vi "Multi U-Link DAQ Single value.vi"() -> ()   [LabVIEW 2017]
uses:
  Type Def/Data.ctl
  <vilib>/Analysis/NI_AALBase.lvlib
panel:
  out "Energie IR mean":dbl caption="moyenne" format="%g"
  out "Energie IR variance":dbl caption="variance" format="%g"
  out "Energie IR max":dbl caption="max" format="%#_5g"
  out "Energie IR min":dbl caption="min"
  out "Puissance depolar mean":dbl caption="moyenne" format="%g"
  out "Puissance depolar variance":dbl caption="variance" format="%g"
  out "Puissance depolar max":dbl caption="max" format="%#_5g"
  out "Puissance depolar min":dbl caption="min" format="%#_5g"
  out "Energie UV mean":dbl caption="moyenne" format="%g"
  out "Energie UV variance":dbl caption="variance" format="%g"
  out "Energie UV max":dbl caption="max" format="%#_5g"
  out "Energie UV min":dbl caption="min" format="%#_5g"
  out "Energie UV rapport":dbl caption="rapport" format="%#_5g"
  out "Puissance depolar rapport":dbl caption="rapport" format="%#_5g"
  out "Energie IR rapport":dbl caption="rapport" format="%#_5g"
  out "Chaîne":string="Energie UV"
  out "Chaîne 2":string="Puissance depolar"
  out "Chaîne 3":string="Energie IR"
  out "sortie d'erreur":errorcluster caption="Sortie d'erreur"
  in  "stop":bool
  out "Energie IR value":dbl format="%#_4f"
  out "Energie IR graph":dbl(graph)
  out "Puissance depolar value":dbl format="%#_4f"
  out "Puissance depolar graph":dbl(graph)
  out "Energie IR table":dbl[](array[numeric])
  out "Energie IR table (1sec)":dbl[](array[numeric])
  out "Puissance depolar table":dbl[](array[numeric])
  out "Energie UV value":dbl format="%#_4f"
  out "Energie UV graph":dbl(graph)
  out "Energie UV table":dbl[](array[numeric])
  out "Energie UV table(1sec)":dbl[](array[numeric])
  out "Taux depolar value":dbl format="%#_4f"
  out "taux depolar graph":dbl(graph)
  out "Puissance depolar table (stats)":dbl[][](array[numeric])
  out "Energie IR table (stats)":dbl[][](array[numeric])
  out "Taux depolar indicator":u32(colorbox)=16777222
  out "Puissance depolar table (1sec)":dbl[](array[numeric])
  out "Energie UV table (stats)":dbl[][](array[numeric])
  out "timer 1sec":bool
  out "timer 12sec":bool
  in  "1sec":bool
  in  "12sec":bool
  out "index 1sec":i32
  out "index 12sec":i32
  out "Chaîne 4":string="Energie UV (mJ)"
  out "Chaîne 5":string="Energie IR (mJ)"
  out "Chaîne 6":string="Puissance depolar (W)"
  out "Chaîne 7":string="Taux depolar"
  out "Update":string="Initialization : matching U-Link ports, creating data file"
  in  "Start acquisition":bool
  in  "Commande onglets":T1(tab)
  out "Ressource VISA (Energie UV)":refnum<visa-resource-name>
  in  "Wavelength (nm) (Energie UV)":u32=355
  in  "Offset (Energie UV)":sgl
  in  "Multiplier (Energie UV)":sgl=1.0
  in  "Trigger Level (% of Scale) (Energie UV)":dbl=2.0 min=0.1 max=99.9 step=0.1 format="%_3f"
  in  "Auto Scale (Energie UV)":bool=TRUE
  out "File name (Energie UV)":string="data.csv"
  in  "Scale (Watt or Joule) (Energie UV)":i32(ring) items=["1 pico", "3 pico", "10 pico", "30 pico", "100 pico", "300 pico", "1 nano", "3 nano", "10 nano", "30 nano", "100 nano", "300 nano", "1 micro", "3 micro", "10 micro", "30 micro", "100 micro", "300 micro", "1 milli", "3 milli", "10 milli", "30 milli", "100 milli", "300 milli", "1", "3", "10", "30", "100", "300", "1 kilo", "3 kilo", "10 kilo", "30 kilo", "100 kilo", "300 kilo", "1 mega", "3 mega", "10 mega", "30 mega", "100 mega", "300 mega"]
  out "Ressource VISA (Puissance depolar)":refnum<visa-resource-name>
  in  "Offset (Puissance depolar)":sgl
  in  "Wavelength (nm) (Puissance depolar)":u32=1064
  in  "Multiplier (Puissance depolar)":sgl=1.0
  in  "Trigger Level (% of Scale) (Puissance depolar)":dbl=2.0 min=0.1 max=99.9 step=0.1 format="%_3f"
  in  "Auto Scale (Puissance depolar)":bool=TRUE
  out "File name (Puissance depolar)":string="data.csv"
  in  "Scale (Watt or Joule) (Puissance depolar)":u16(ring) items=["1 pico", "3 pico", "10 pico", "30 pico", "100 pico", "300 pico", "1 nano", "3 nano", "10 nano", "30 nano", "100 nano", "300 nano", "1 micro", "3 micro", "10 micro", "30 micro", "100 micro", "300 micro", "1 milli", "3 milli", "10 milli", "30 milli", "100 milli", "300 milli", "1", "3", "10", "30", "100", "300", "1 kilo", "3 kilo", "10 kilo", "30 kilo", "100 kilo", "300 kilo", "1 mega", "3 mega", "10 mega", "30 mega", "100 mega", "300 mega"]
  out "Ressource VISA (Energie IR)":refnum<visa-resource-name>
  in  "Wavelength (nm) (Energie IR)":u32=1064
  in  "Offset (Energie IR)":sgl
  in  "Multiplier (Energie IR)":sgl=1.0
  in  "Trigger Level (% of Scale) (Energie IR)":dbl=2.0 min=0.1 max=99.9 step=0.1 format="%_3f"
  out "File name (Energie IR)":string="data.csv"
  in  "Scale (Watt or Joule) (Energie IR)":u16(ring) items=["1 pico", "3 pico", "10 pico", "30 pico", "100 pico", "300 pico", "1 nano", "3 nano", "10 nano", "30 nano", "100 nano", "300 nano", "1 micro", "3 micro", "10 micro", "30 micro", "100 micro", "300 micro", "1 milli", "3 milli", "10 milli", "30 milli", "100 milli", "300 milli", "1", "3", "10", "30", "100", "300", "1 kilo", "3 kilo", "10 kilo", "30 kilo", "100 kilo", "300 kilo", "1 mega", "3 mega", "10 mega", "30 mega", "100 mega", "300 mega"]
  in  "Auto Scale (Energie IR)":bool
  out "error IO":errorcluster
  out "COM Port table":refnum<visa-resource-name>[](array[refnum])
  out "COM Port (Energie IR)":i64
  out "COM Port (Puissance depolar)":i64
  out "COM port (Energie UV)":i64
  out "User file contents Energie UV":dbl[](array[numeric])
  out "User file contents Energie IR":dbl[](array[numeric])
  out "User file contents Puissance depolar":dbl[](array[numeric])
  out "error?":bool caption="erreur ?"
  out "file path":path
  out "sortie d'erreur 3":errorcluster caption="sortie d'erreur"
  out "sortie d'erreur 2":errorcluster caption="sortie d'erreur"
  out "Energie UV file (1sec)":refnum<file>
  out "Energie UV file (stats)":refnum<file>
  out "Puissance depolar file (1sec)":refnum<file>
  out "Puissance depolar file (stats)":refnum<file>
  out "Energie IR file (1sec)":refnum<file>
  out "Energie IR file (stats)":refnum<file>
  in  "Bouton Accueil":bool
  out "chaîne de date/heure":string
  out "valeur de l'horloge en ms":u32
  out "Time":string
  out "stop?":bool=TRUE
  out "Tableau Puissance depolar":dbl[](array[numeric])
  out "Tableau UV":dbl[](array[numeric])
  out "Tableau IR":dbl[](array[numeric])
  out "taille UV":dbl format="%.2f"
  out "taille Pd":dbl format="%.2f"
  out "taille IR":dbl format="%.2f"
  out "12sec UV":bool
  out "12sec Pd":bool
  out "12sec IR":bool
  out "stop UV":bool
  out "stop Pd":bool
  out "stop IR":bool
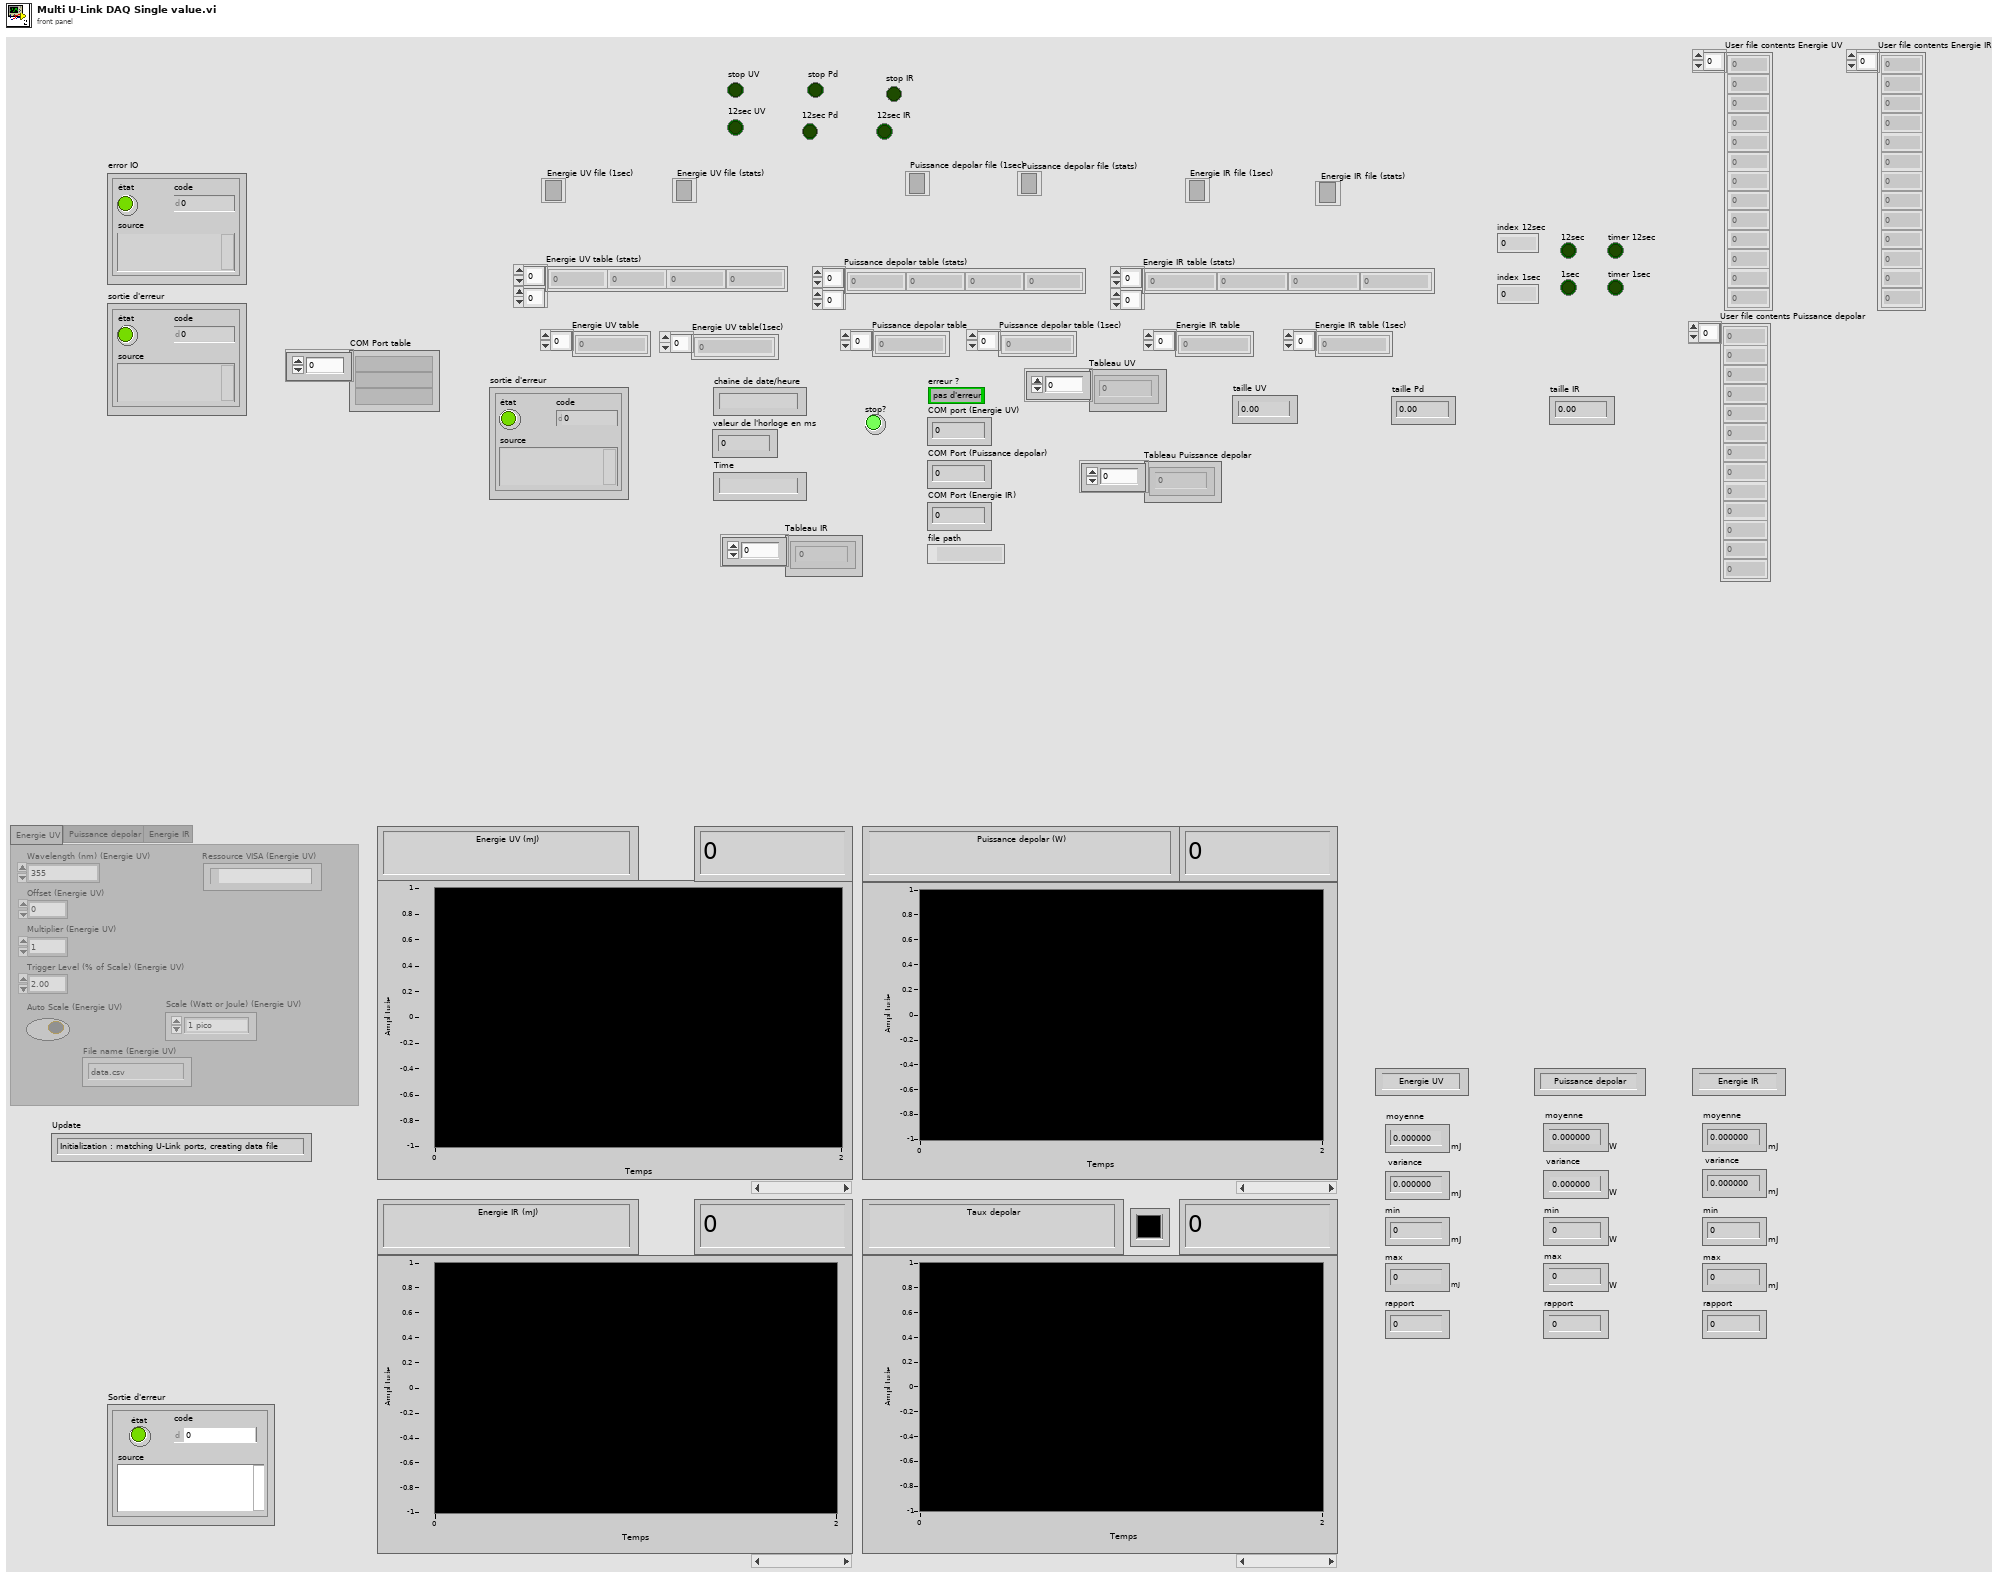
[diagram p1: front panel]
types:
  T1 = enum32{"Energie UV", "Puissance depolar", "Energie IR"}
  T2 = enum8{"Enabled", "Disabled", "Disabled and Grayed Out"}
  T3 = typedef "Data.ctl" = cluster{enum16{"Init", "Read", "Stop", "12sec"}, "Data":dbl}
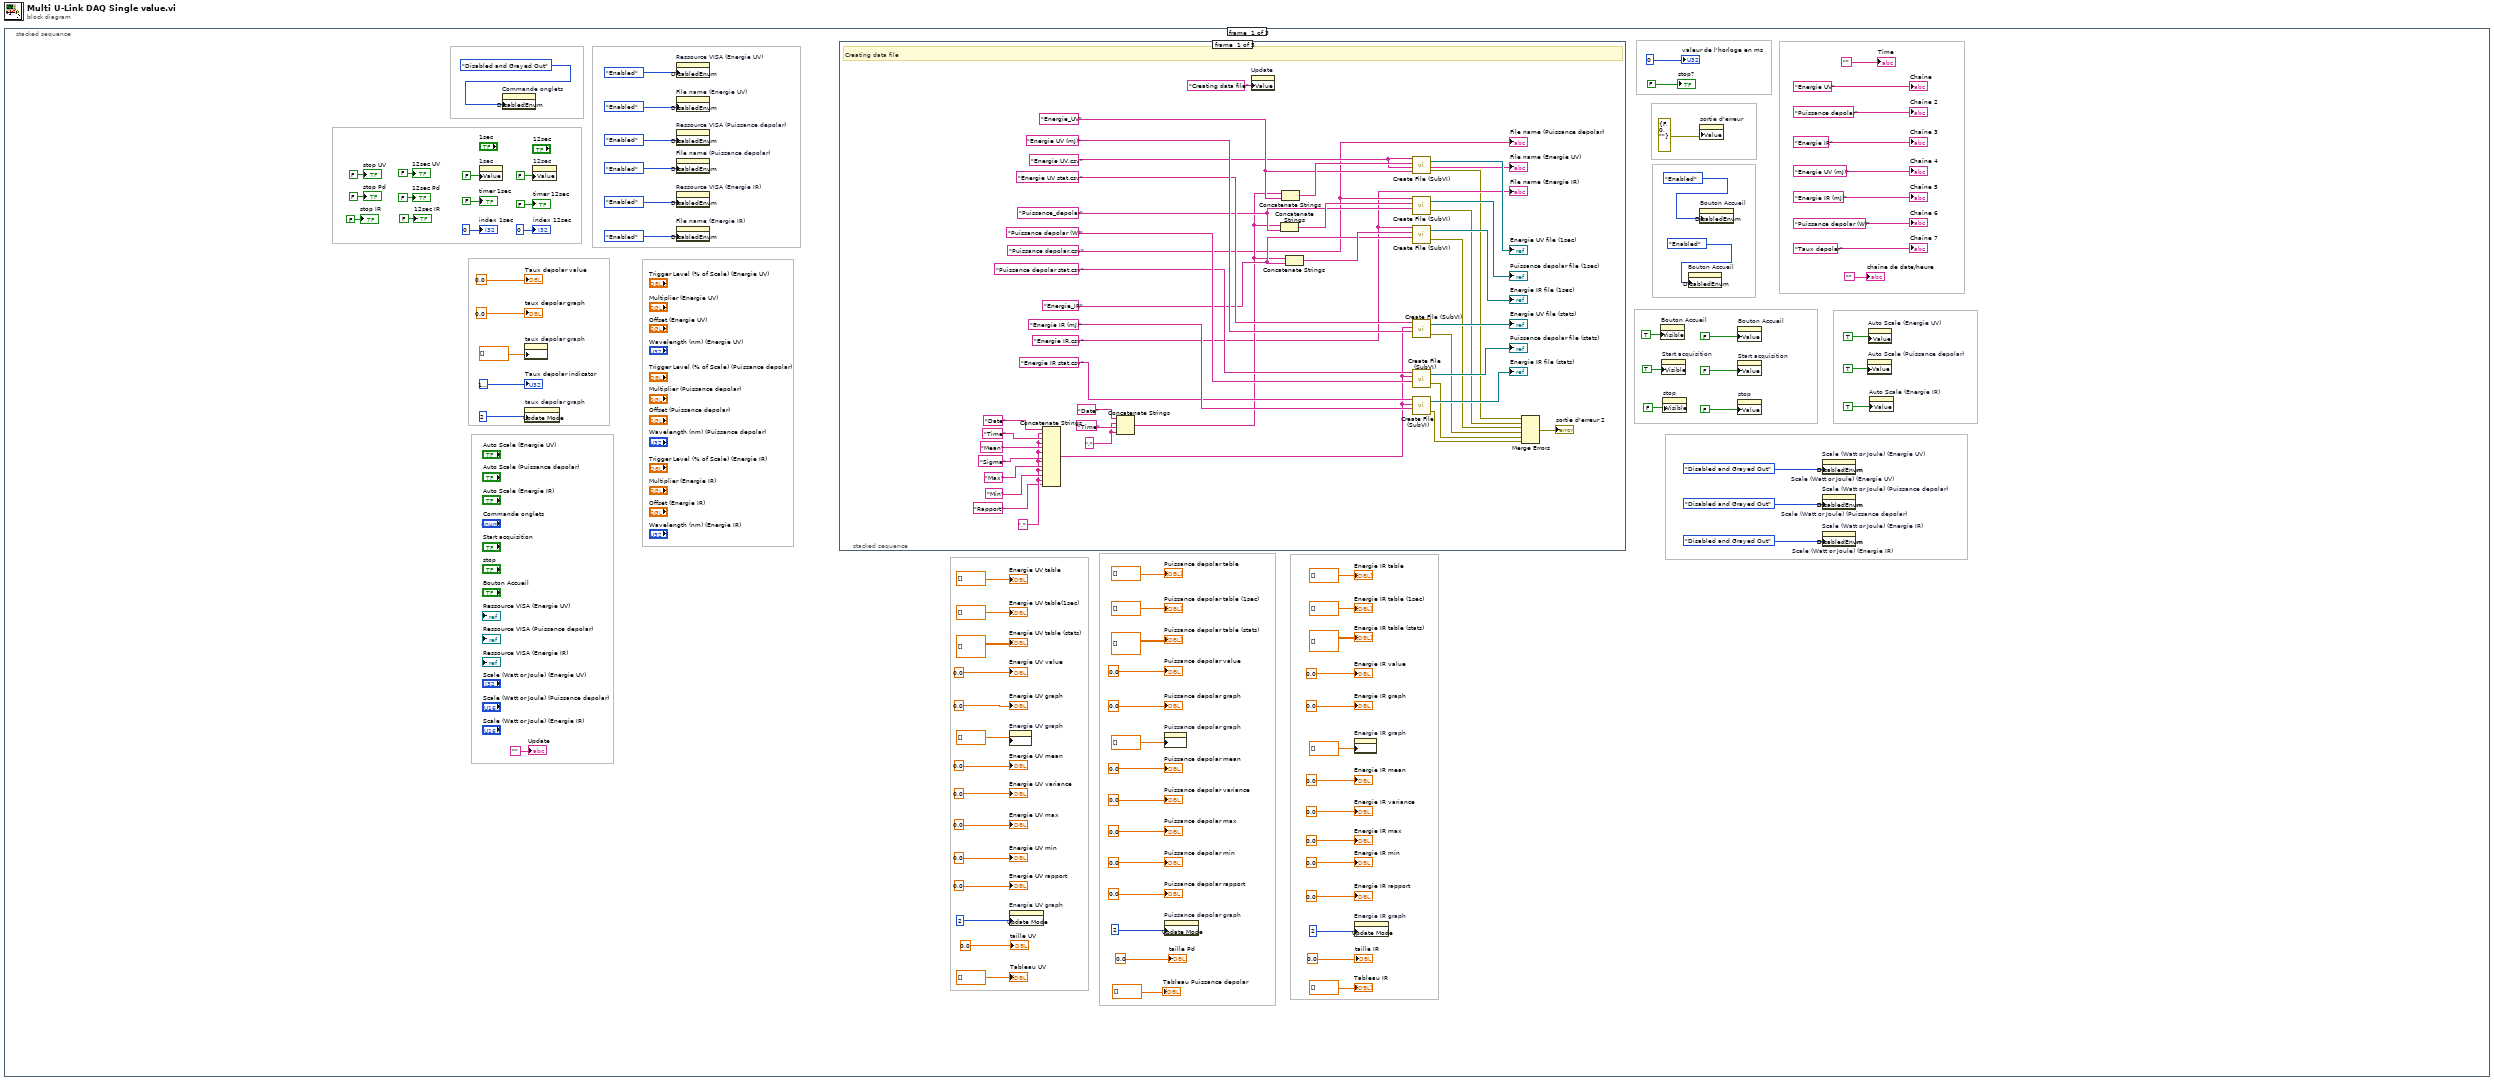
[diagram p0: block diagram]
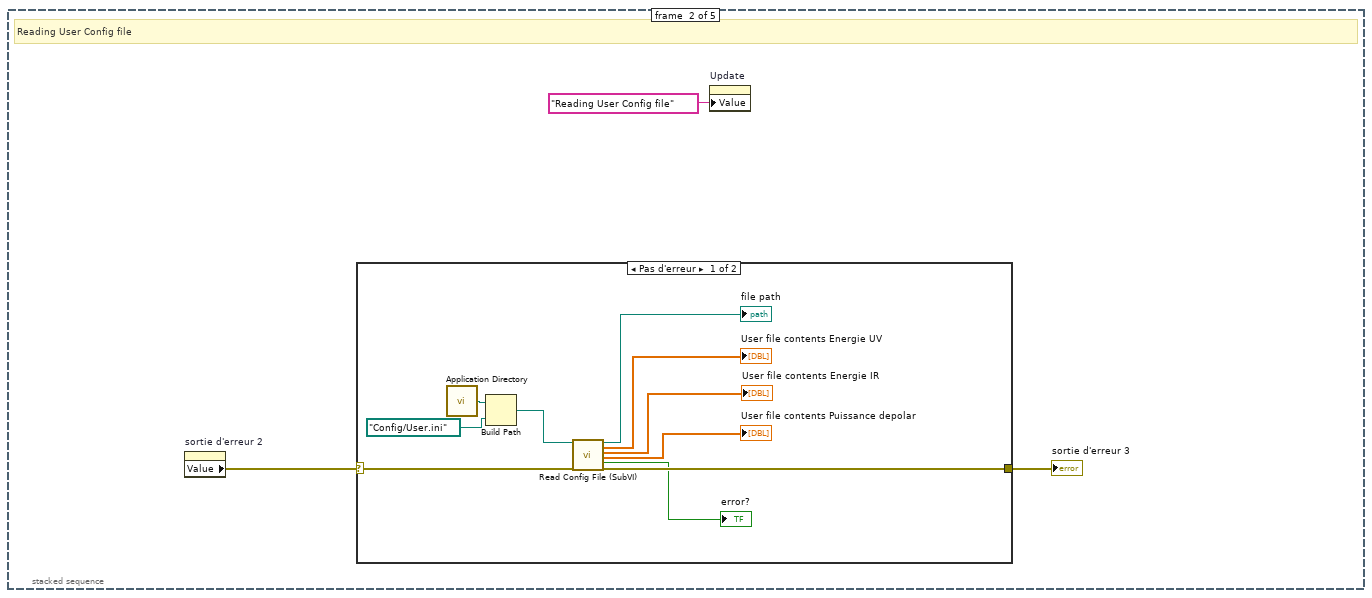
[diagram p2: hidden frame]
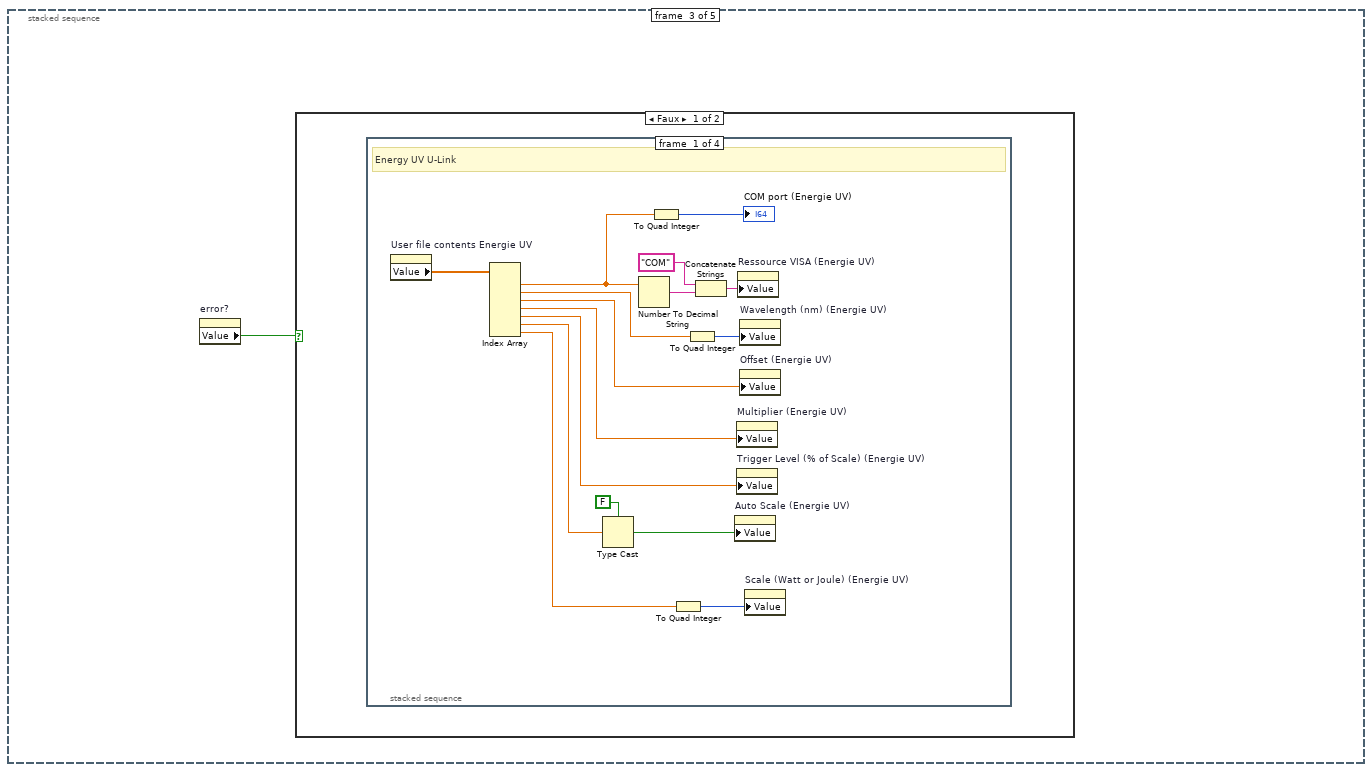
[diagram p4: hidden frame]
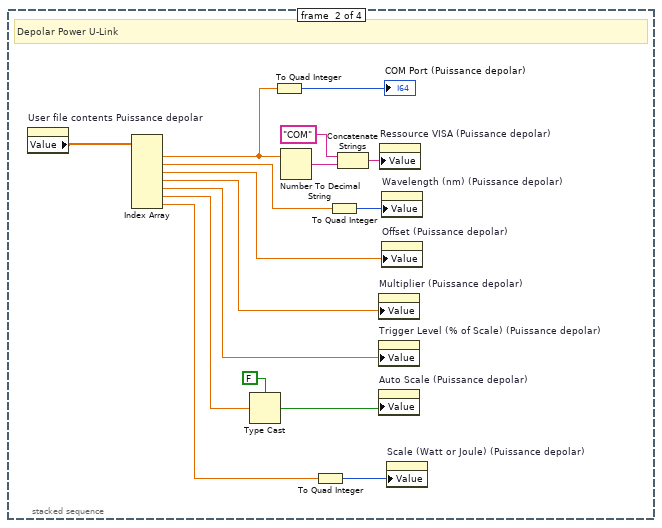
[diagram p5: hidden frame]
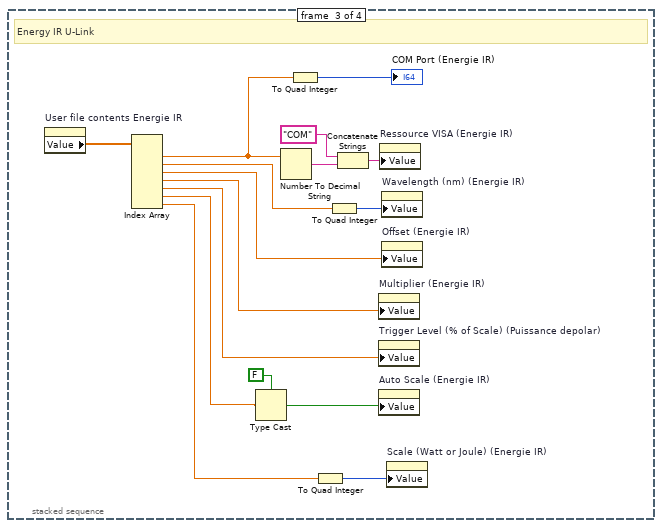
[diagram p6: hidden frame]
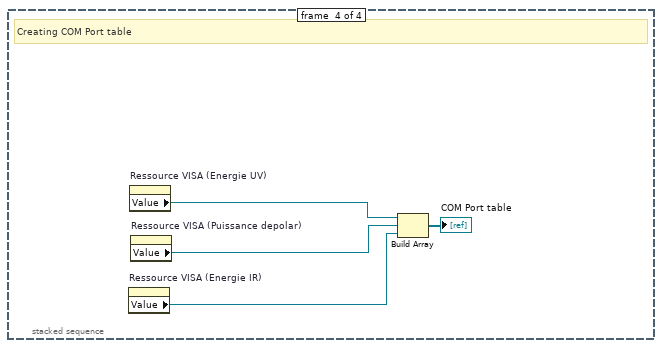
[diagram p7: hidden frame]
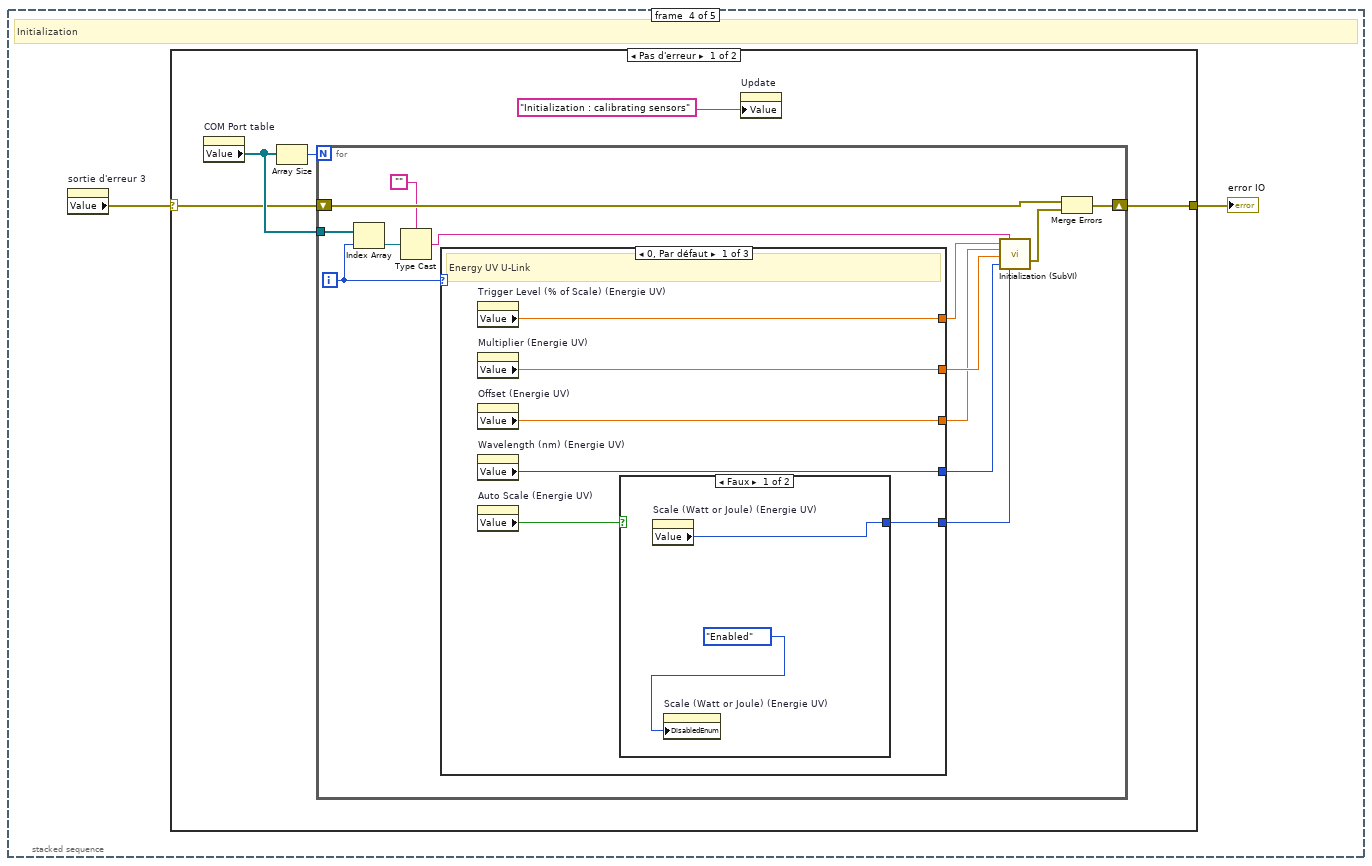
[diagram p9: hidden frame]
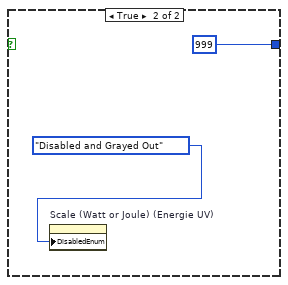
[diagram p10: hidden frame]
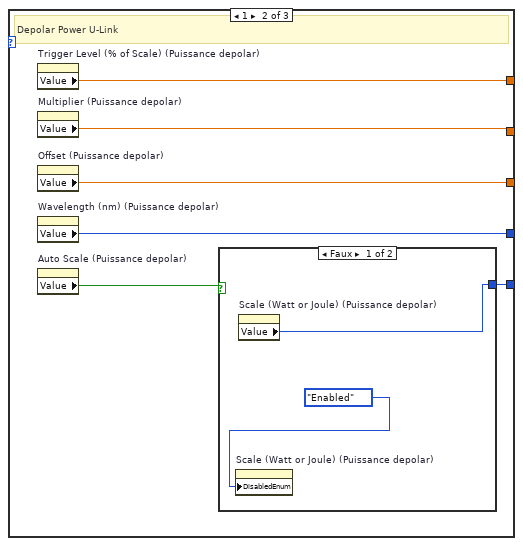
[diagram p11: hidden frame]
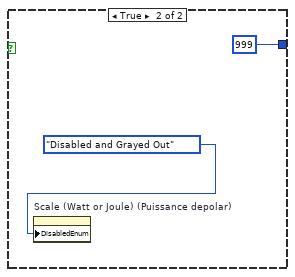
[diagram p12: hidden frame]
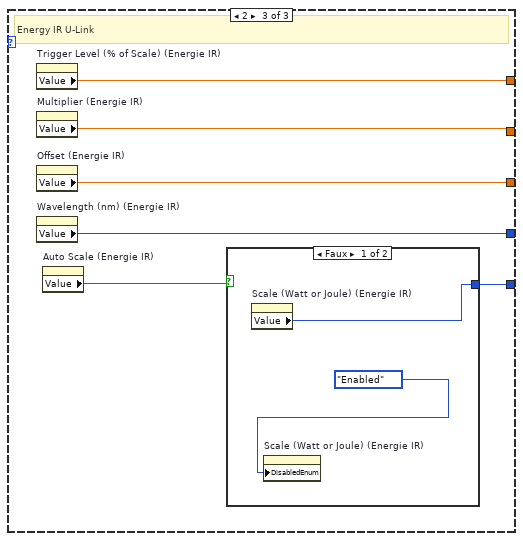
[diagram p13: hidden frame]
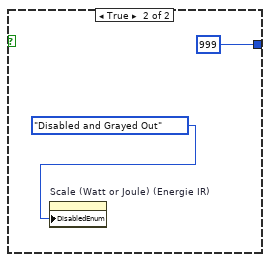
[diagram p14: hidden frame]
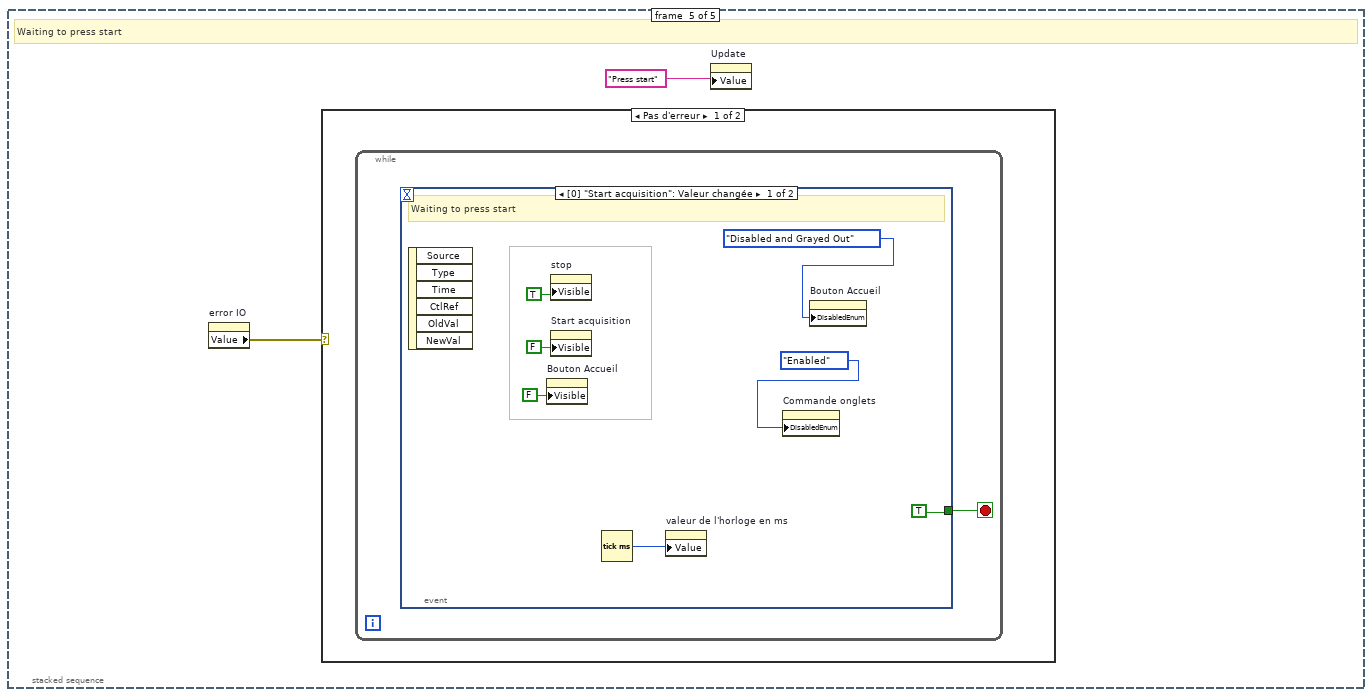
[diagram p16: hidden frame]
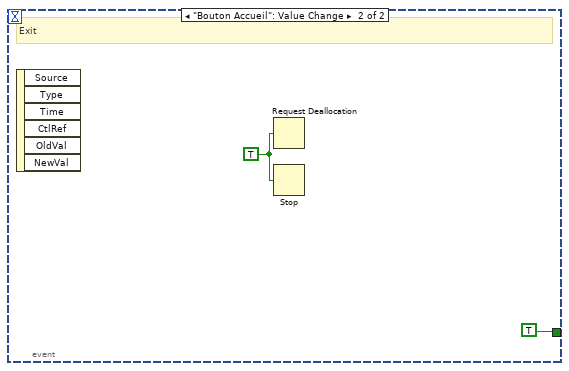
[diagram p17: hidden frame]
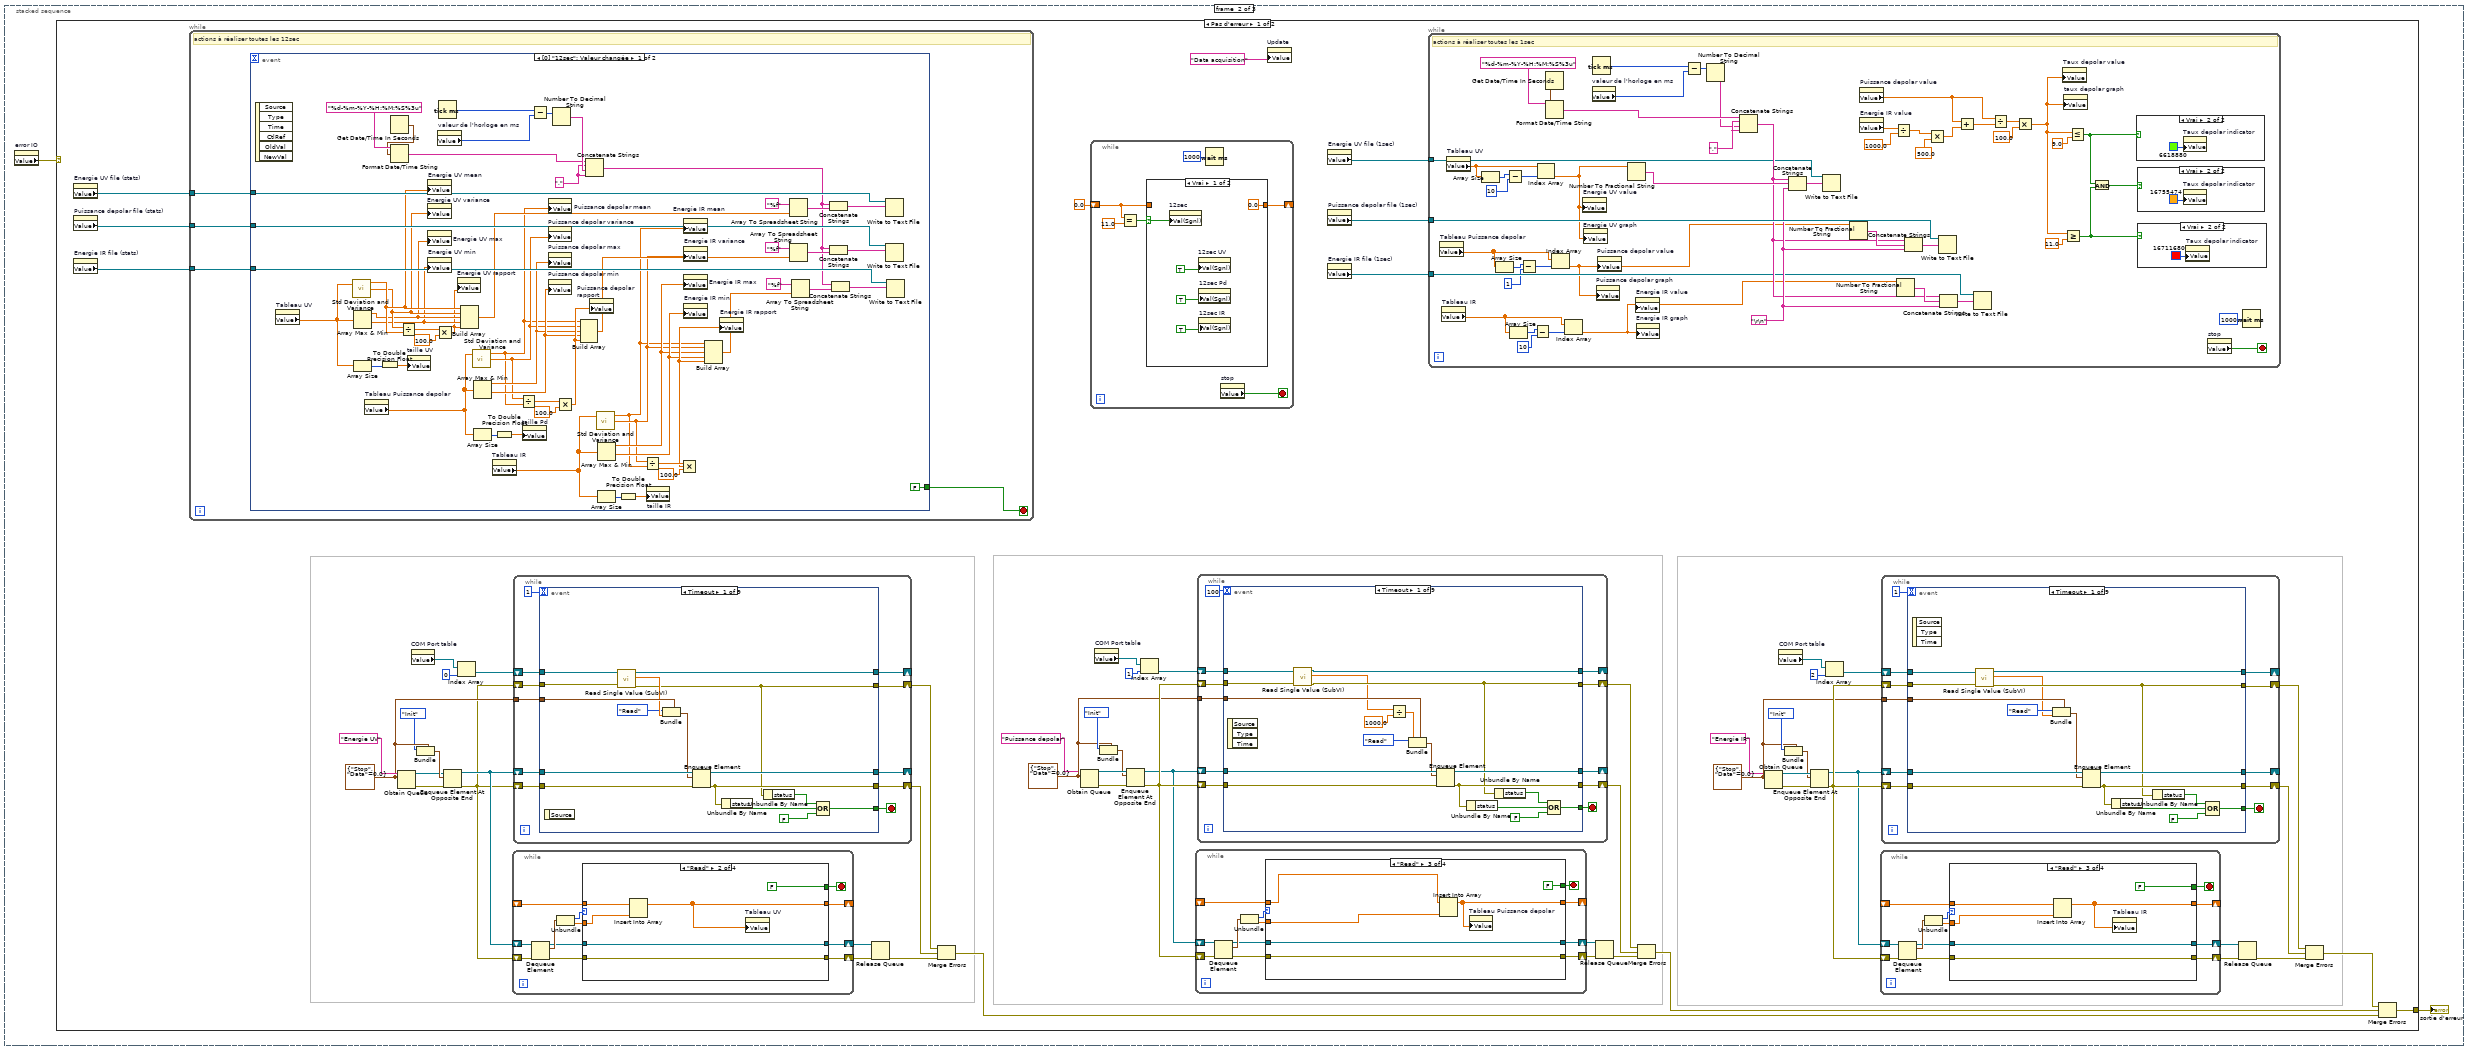
[diagram p19: hidden frame]
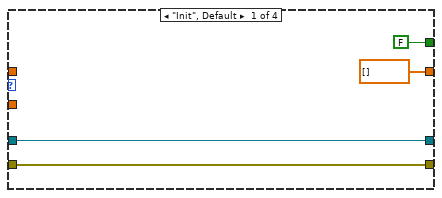
[diagram p20: hidden frame]
diagram:
  n1 = stacked-sequence {
    frame #0 {
      n2 = property on="1sec" class="Bool (strict)"("Value"=FALSE ("1sec")) -> ()  [unwired: 2 in, 2 out]
      n3 = property on="Commande onglets" class="Onglet (strict)"("DisabledEnum"=T2."Disabled and Grayed Out" ("Désactivé")) -> ()  [unwired: 2 in, 2 out]
      n4 = property on="taux depolar graph" class="GraphDér (strict)"("History Data"=dbl[] [] ("Données d'historique")) -> ()  [unwired: 2 in, 2 out]
      n5 = property on="taux depolar graph" class="GraphDér (strict)"("Update Mode"=u8 2 ("Mode de rafraîchissement")) -> ()  [unwired: 2 in, 2 out]
      n6 = property on="12sec" class="Bool (strict)"("Value"=FALSE ("12sec")) -> ()  [unwired: 2 in, 2 out]
      n7 = property on="Ressource VISA (Energie UV)" class="NomVISA"("DisabledEnum"=T2."Enabled" ("Désactivé")) -> ()  [unwired: 2 in, 2 out]
      n8 = property on="File name (Energie UV)" class="Ch"("DisabledEnum"=T2."Enabled" ("Désactivé")) -> ()  [unwired: 2 in, 2 out]
      n9 = property on="Ressource VISA (Puissance depolar)" class="NomVISA"("DisabledEnum"=T2."Enabled" ("Désactivé")) -> ()  [unwired: 2 in, 2 out]
      n10 = property on="File name (Puissance depolar)" class="Ch"("DisabledEnum"=T2."Enabled" ("Désactivé")) -> ()  [unwired: 2 in, 2 out]
      n11 = property on="Ressource VISA (Energie IR)" class="NomVISA"("DisabledEnum"=T2."Enabled" ("Désactivé")) -> ()  [unwired: 2 in, 2 out]
      n12 = property on="File name (Energie IR)" class="Ch"("DisabledEnum"=T2."Enabled" ("Désactivé")) -> ()  [unwired: 2 in, 2 out]
      n13 = stacked-sequence {
        frame #0 {
          w114 = ","
          w104 = ","
          w105 = "Energie IR.csv" ("file name 2")
          w109 = "Energie_IR" ("data name")
          w106 = "Puissance depolar.csv" ("file name 2")
          w111 = "Puissance_depolar" ("data name")
          w107 = "Energie UV.csv" ("file name")
          w116 = "Energie_UV" ("data name")
          # "Creating data file"
          n14 = Concatenate Strings("Date", w104, "Time", w104, "Mean", w104, "Sigma", w104, "Max", w104, "Min", w104, "Rapport" ("chaîne")) -> (w120:string)
          n15 = Concatenate Strings("Date", w114, "Time", w114) -> (w108:string)
          n16 = property on="Update" class="Ch"("Value"="Creating data file" ("Étiquette.Texte")) -> ()  [unwired: 2 in, 2 out]
          n17 = Concatenate Strings(w108, w111) -> (w112:string)
          n18 = Concatenate Strings(w108, w116) -> (w117:string)
          n19 = Concatenate Strings(w108, w109) -> (w110:string)
          n20 = call "Create File (SubVI).vi"("headers"=w116, "data name"=w117, "file name"=w107) -> ("error out"=w97:errorcluster, "Byte Stream File out"=→"Energie UV file (1sec)":refnum<file>)  [unwired: 1 in]
          n21 = call "Create File (SubVI).vi"("headers"=w111, "data name"=w112, "file name"=w106) -> ("error out"=w98:errorcluster, "Byte Stream File out"=→"Puissance depolar file (1sec)":refnum<file>)  [unwired: 1 in]
          n22 = call "Create File (SubVI).vi"("headers"=w109, "data name"=w110, "file name"=w105) -> ("error out"=w99:errorcluster, "Byte Stream File out"=→"Energie IR file (1sec)":refnum<file>)  [unwired: 1 in]
          n23 = call "Create File (SubVI).vi"("headers"="Energie UV (mJ)" ("data name"), "data name"=w120, "file name"="Energie UV stat.csv") -> ("error out"=w100:errorcluster, "Byte Stream File out"=→"Energie UV file (stats)":refnum<file>)  [unwired: 1 in]
          n24 = call "Create File (SubVI).vi"("headers"="Puissance depolar (W)" ("data name"), "data name"=w120, "file name"="Puissance depolar stat.csv" ("file name 2")) -> ("error out"=w101:errorcluster, "Byte Stream File out"=→"Puissance depolar file (stats)":refnum<file>)  [unwired: 1 in]
          n25 = call "Create File (SubVI).vi"("headers"="Energie IR (mJ)" ("data name"), "data name"=w120, "file name"="Energie IR stat.csv" ("file name 2")) -> ("error out"=w102:errorcluster, "Byte Stream File out"=→"Energie IR file (stats)":refnum<file>)  [unwired: 1 in]
          n26 = Merge Errors(w97, w98, w99, w100, w101, w102) -> (→"sortie d'erreur 2":errorcluster)
          "File name (Energie UV)" <- w107
          "File name (Puissance depolar)" <- w106
          "File name (Energie IR)" <- w105
        }
        frame #1 {
          # "Reading User Config file"
          n27 = property on="sortie d'erreur 2" class="Clust (strict)"() -> ("Value"=w141:errorcluster)  [unwired: 2 in, 2 out]
          n28 = case shown="Pas d'erreur" w141 {
            selector: w141 -> [w150 w152]
            tunnel: [w151 w152] -> w140
            frame No Error {
              n29 = call <vilib>:"Application Directory.vi"() -> ("Application Directory"=w146:path)
              n30 = Build Path(base path=w146, name or relative path=path "Config/User.ini") -> (appended path=w144:path)
              n31 = call "Read Config File (SubVI).vi"("configuration file path"=w144, "entrée d'erreur (pas d'erreur)"=w150) -> ("file path"=→"file path":path, "User file contents Energie UV"=→"User file contents Energie UV":dbl[], "User file contents Energie IR"=→"User file contents Energie IR":dbl[], "User file contents Puissance depolar"=→"User file contents Puissance depolar":dbl[], "error?"=→"error?":bool, "sortie d'erreur"=w151:errorcluster)  [unwired: 12 in]
            }
            frame Error {
            }
          }
          "sortie d'erreur 3" <- w140
          n32 = property on="Update" class="Ch"("Value"="Reading User Config file" ("Étiquette.Texte")) -> ()  [unwired: 2 in, 2 out]
        }
        frame #2 {
          n33 = property on="error?" class="Bool (strict)"() -> ("Value"=w153:bool)  [unwired: 2 in, 2 out]
          n34 = case shown="Faux" w153 {
            frame False {
              n35 = stacked-sequence {
                frame #0 {
                  # "Energy UV U-Link"
                  n36 = property on="User file contents Energie UV" class="Tabl (strict)"() -> ("Value"=w154:dbl[])  [unwired: 2 in, 2 out]
                  n37 = Index Array(array=w154) -> (element #1=w166:dbl, element #2=w165:dbl, element #3=w163:dbl, element #4=w162:dbl, element #5=w157:dbl, element #6=w156:dbl, element #7=w155:dbl)  [unwired: 7 in]
                  n38 = Type Cast(type=FALSE, x=w156) -> (*(type *) &x=w159:bool)
                  n39 = Number To Decimal String(number=w166) -> (decimal integer string=w168:string)  [unwired: 1 in]
                  n40 = To Quad Integer(1:w166) -> (0:→"COM port (Energie UV)":i64)
                  n41 = To Quad Integer(1:w155) -> (0:w161:i64)
                  n42 = To Quad Integer(1:w165) -> (0:w164:i64)
                  n43 = Concatenate Strings("COM" ("string"), w168) -> (w167:string)
                  n44 = property on="Auto Scale (Energie UV)" class="Bool (strict)"("Value"=w159) -> ()  [unwired: 2 in, 2 out]
                  n45 = property on="Multiplier (Energie UV)" class="NumNb (strict)"("Value"=w162) -> ()  [unwired: 2 in, 2 out]
                  n46 = property on="Trigger Level (% of Scale) (Energie UV)" class="NumNb (strict)"("Value"=w157) -> ()  [unwired: 2 in, 2 out]
                  n47 = property on="Ressource VISA (Energie UV)" class="NomVISA"("Value"=w167) -> ()  [unwired: 2 in, 2 out]
                  n48 = property on="Wavelength (nm) (Energie UV)" class="NumNb (strict)"("Value"=w164) -> ()  [unwired: 2 in, 2 out]
                  n49 = property on="Offset (Energie UV)" class="NumNb (strict)"("Value"=w163) -> ()  [unwired: 2 in, 2 out]
                  n50 = property on="Scale (Watt or Joule) (Energie UV)" class="MDér (strict)"("Value"=w161) -> ()  [unwired: 2 in, 2 out]
                }
                frame #1 {
                  # "Depolar Power U-Link"
                  n51 = property on="User file contents Puissance depolar" class="Tabl (strict)"() -> ("Value"=w176:dbl[])  [unwired: 2 in, 2 out]
                  n52 = Index Array(array=w176) -> (element #1=w182:dbl, element #2=w181:dbl, element #3=w179:dbl, element #4=w178:dbl, element #5=w172:dbl, element #6=w171:dbl, element #7=w170:dbl)  [unwired: 7 in]
                  n53 = Type Cast(type=FALSE, x=w171) -> (*(type *) &x=w173:bool)
                  n54 = To Quad Integer(1:w182) -> (0:→"COM Port (Puissance depolar)":i64)
                  n55 = Number To Decimal String(number=w182) -> (decimal integer string=w184:string)  [unwired: 1 in]
                  n56 = To Quad Integer(1:w170) -> (0:w177:i64)
                  n57 = To Quad Integer(1:w181) -> (0:w180:i64)
                  n58 = Concatenate Strings("COM" ("string"), w184) -> (w183:string)
                  n59 = property on="Multiplier (Puissance depolar)" class="NumNb (strict)"("Value"=w178) -> ()  [unwired: 2 in, 2 out]
                  n60 = property on="Trigger Level (% of Scale) (Puissance depolar)" class="NumNb (strict)"("Value"=w172) -> ()  [unwired: 2 in, 2 out]
                  n61 = property on="Auto Scale (Puissance depolar)" class="Bool (strict)"("Value"=w173) -> ()  [unwired: 2 in, 2 out]
                  n62 = property on="Ressource VISA (Puissance depolar)" class="NomVISA"("Value"=w183) -> ()  [unwired: 2 in, 2 out]
                  n63 = property on="Wavelength (nm) (Puissance depolar)" class="NumNb (strict)"("Value"=w180) -> ()  [unwired: 2 in, 2 out]
                  n64 = property on="Offset (Puissance depolar)" class="NumNb (strict)"("Value"=w179) -> ()  [unwired: 2 in, 2 out]
                  n65 = property on="Scale (Watt or Joule) (Puissance depolar)" class="MDér (strict)"("Value"=w177) -> ()  [unwired: 2 in, 2 out]
                }
                frame #2 {
                  # "Energy IR U-Link"
                  n66 = property on="User file contents Energie IR" class="Tabl (strict)"() -> ("Value"=w192:dbl[])  [unwired: 2 in, 2 out]
                  n67 = Index Array(array=w192) -> (element #1=w198:dbl, element #2=w197:dbl, element #3=w195:dbl, element #4=w194:dbl, element #5=w188:dbl, element #6=w187:dbl, element #7=w186:dbl)  [unwired: 7 in]
                  n68 = Type Cast(type=FALSE, x=w187) -> (*(type *) &x=w190:bool)
                  n69 = Number To Decimal String(number=w198) -> (decimal integer string=w200:string)  [unwired: 1 in]
                  n70 = To Quad Integer(1:w198) -> (0:→"COM Port (Energie IR)":i64)
                  n71 = To Quad Integer(1:w186) -> (0:w193:i64)
                  n72 = To Quad Integer(1:w197) -> (0:w196:i64)
                  n73 = Concatenate Strings("COM" ("string"), w200) -> (w199:string)
                  n74 = property on="Multiplier (Energie IR)" class="NumNb (strict)"("Value"=w194) -> ()  [unwired: 2 in, 2 out]
                  n75 = property on="Trigger Level (% of Scale) (Puissance depolar)" class="NumNb (strict)"("Value"=w188) -> ()  [unwired: 2 in, 2 out]
                  n76 = property on="Auto Scale (Energie IR)" class="Bool (strict)"("Value"=w190) -> ()  [unwired: 2 in, 2 out]
                  n77 = property on="Ressource VISA (Energie IR)" class="NomVISA"("Value"=w199) -> ()  [unwired: 2 in, 2 out]
                  n78 = property on="Wavelength (nm) (Energie IR)" class="NumNb (strict)"("Value"=w196) -> ()  [unwired: 2 in, 2 out]
                  n79 = property on="Offset (Energie IR)" class="NumNb (strict)"("Value"=w195) -> ()  [unwired: 2 in, 2 out]
                  n80 = property on="Scale (Watt or Joule) (Energie IR)" class="MDér (strict)"("Value"=w193) -> ()  [unwired: 2 in, 2 out]
                }
                frame #3 {
                  # "Creating COM Port table"
                  n81 = property on="Ressource VISA (Energie IR)" class="NomVISA"() -> ("Value"=w205:refnum<visa-resource-name>)  [unwired: 2 in, 2 out]
                  n82 = property on="Ressource VISA (Energie UV)" class="NomVISA"() -> ("Value"=w203:refnum<visa-resource-name>)  [unwired: 2 in, 2 out]
                  n83 = property on="Ressource VISA (Puissance depolar)" class="NomVISA"() -> ("Value"=w204:refnum<visa-resource-name>)  [unwired: 2 in, 2 out]
                  n84 = Build Array(w203, w204, w205) -> (→"COM Port table":refnum<visa-resource-name>[])
                }
              }
            }
            frame True {
            }
          }
        }
        frame #3 {
          # "Initialization"
          n85 = property on="sortie d'erreur 3" class="Clust (strict)"() -> ("Value"=w206:errorcluster)  [unwired: 2 in, 2 out]
          n86 = case shown="Pas d'erreur" w206 {
            selector: w206 -> [w208 w256]
            tunnel: [w211 w256] -> w207
            frame No Error {
              n87 = property on="COM Port table" class="Tabl (strict)"() -> ("Value"=w209:refnum<visa-resource-name>[])  [unwired: 2 in, 2 out]
              n88 = Array Size(array=w209) -> (size(s)=w210:i32)
              n89 = for {
                N: w210 -> [_]
                shift-right: [w219] -> w211
                shift-left: w208 -> [w218]
                tunnel: w209 -> [w213]
                i -> [w214]
                n90 = Index Array(array=w213, index=w214) -> (element=w216:refnum<visa-resource-name>)
                n91 = Type Cast(type="", x=w216) -> (*(type *) &x=w217:string)
                n92 = case shown="0, Par défaut" w214 {
                  tunnel: [w231 w238 w248] -> w225
                  tunnel: [w228 w239 w249] -> w223
                  tunnel: [w230 w240 w250] -> w224
                  tunnel: [w229 w241 w251] -> w222
                  tunnel: [w227 w237 w247] -> w221
                  frame 0, Default {
                    # "Energy UV U-Link"
                    n93 = property on="Trigger Level (% of Scale) (Energie UV)" class="NumNb (strict)"() -> ("Value"=w229:dbl)  [unwired: 2 in, 2 out]
                    n94 = property on="Multiplier (Energie UV)" class="NumNb (strict)"() -> ("Value"=w230:sgl)  [unwired: 2 in, 2 out]
                    n95 = property on="Offset (Energie UV)" class="NumNb (strict)"() -> ("Value"=w228:sgl)  [unwired: 2 in, 2 out]
                    n96 = property on="Wavelength (nm) (Energie UV)" class="NumNb (strict)"() -> ("Value"=w231:u32)  [unwired: 2 in, 2 out]
                    n97 = property on="Auto Scale (Energie UV)" class="Bool (strict)"() -> ("Value"=w226:bool)  [unwired: 2 in, 2 out]
                    n98 = case shown="Faux" w226 {
                      tunnel: [w233 u32 999 ("Value")] -> w227
                      frame False {
                        n99 = property on="Scale (Watt or Joule) (Energie UV)" class="MDér (strict)"() -> ("Value"=w233:i32)  [unwired: 2 in, 2 out]
                        n100 = property on="Scale (Watt or Joule) (Energie UV)" class="MDér (strict)"("DisabledEnum"=T2."Enabled" ("Désactivé")) -> ()  [unwired: 2 in, 2 out]
                      }
                      frame True {
                        n101 = property on="Scale (Watt or Joule) (Energie UV)" class="MDér (strict)"("DisabledEnum"=T2."Disabled and Grayed Out" ("Désactivé")) -> ()  [unwired: 2 in, 2 out]
                      }
                    }
                  }
                  frame 1 {
                    # "Depolar Power U-Link"
                    n102 = property on="Trigger Level (% of Scale) (Puissance depolar)" class="NumNb (strict)"() -> ("Value"=w241:dbl)  [unwired: 2 in, 2 out]
                    n103 = property on="Multiplier (Puissance depolar)" class="NumNb (strict)"() -> ("Value"=w240:sgl)  [unwired: 2 in, 2 out]
                    n104 = property on="Offset (Puissance depolar)" class="NumNb (strict)"() -> ("Value"=w239:sgl)  [unwired: 2 in, 2 out]
                    n105 = property on="Wavelength (nm) (Puissance depolar)" class="NumNb (strict)"() -> ("Value"=w238:u32)  [unwired: 2 in, 2 out]
                    n106 = property on="Auto Scale (Puissance depolar)" class="Bool (strict)"() -> ("Value"=w236:bool)  [unwired: 2 in, 2 out]
                    n107 = case shown="Faux" w236 {
                      tunnel: [w243 u32 999 ("Value")] -> w237
                      frame False {
                        n108 = property on="Scale (Watt or Joule) (Puissance depolar)" class="MDér (strict)"("DisabledEnum"=T2."Enabled" ("Désactivé")) -> ()  [unwired: 2 in, 2 out]
                        n109 = property on="Scale (Watt or Joule) (Puissance depolar)" class="MDér (strict)"() -> ("Value"=w243:u16)  [unwired: 2 in, 2 out]
                      }
                      frame True {
                        n110 = property on="Scale (Watt or Joule) (Puissance depolar)" class="MDér (strict)"("DisabledEnum"=T2."Disabled and Grayed Out" ("Désactivé")) -> ()  [unwired: 2 in, 2 out]
                      }
                    }
                  }
                  frame 2 {
                    # "Energy IR U-Link"
                    n111 = property on="Trigger Level (% of Scale) (Energie IR)" class="NumNb (strict)"() -> ("Value"=w251:dbl)  [unwired: 2 in, 2 out]
                    n112 = property on="Multiplier (Energie IR)" class="NumNb (strict)"() -> ("Value"=w250:sgl)  [unwired: 2 in, 2 out]
                    n113 = property on="Offset (Energie IR)" class="NumNb (strict)"() -> ("Value"=w249:sgl)  [unwired: 2 in, 2 out]
                    n114 = property on="Wavelength (nm) (Energie IR)" class="NumNb (strict)"() -> ("Value"=w248:u32)  [unwired: 2 in, 2 out]
                    n115 = property on="Auto Scale (Energie IR)" class="Bool (strict)"() -> ("Value"=w246:bool)  [unwired: 2 in, 2 out]
                    n116 = case shown="Faux" w246 {
                      tunnel: [w253 u32 999 ("Value")] -> w247
                      frame False {
                        n117 = property on="Scale (Watt or Joule) (Energie IR)" class="MDér (strict)"() -> ("Value"=w253:u16)  [unwired: 2 in, 2 out]
                        n118 = property on="Scale (Watt or Joule) (Energie IR)" class="MDér (strict)"("DisabledEnum"=T2."Enabled" ("Désactivé")) -> ()  [unwired: 2 in, 2 out]
                      }
                      frame True {
                        n119 = property on="Scale (Watt or Joule) (Energie IR)" class="MDér (strict)"("DisabledEnum"=T2."Disabled and Grayed Out" ("Désactivé")) -> ()  [unwired: 2 in, 2 out]
                      }
                    }
                  }
                }
                n120 = call "Initialization (SubVI).vi"("Trigger Level (% of Scale)"=w222, "VISA Refnum in"=w217, "Offset"=w223, "Multiplier"=w224, "Wavelength (nm)"=w225, "Scale"=w221) -> ("error out"=w220:errorcluster)  [unwired: 8 in, 1 out]
                n121 = Merge Errors(w218, w220) -> (w219:errorcluster)
              }
              n122 = property on="Update" class="Ch"("Value"="Initialization : calibrating sensors" ("Étiquette.Texte")) -> ()  [unwired: 2 in, 2 out]
            }
            frame Error {
            }
          }
          "error IO" <- w207
        }
        frame #4 {
          # "Waiting to press start"
          n123 = property on="error IO" class="Clust (strict)"() -> ("Value"=w258:errorcluster)  [unwired: 2 in, 2 out]
          n124 = case shown="Pas d'erreur" w258 {
            frame No Error {
              n125 = while {
                stop <- w259 stop-if-true
                n126 = event "Structure Événement" shown="[0] \"Start acquisition\": Valeur changée" {
                  selector: _ -> [_ _]
                  dyn-events: _ -> [_ _]
                  timeout: _ -> [_ _]
                  tunnel: [TRUE TRUE] -> w259
                  event "Start acquisition": Value Change {
                    # "Waiting to press start"
                    n127 = event-data() -> ()  [unwired: 1 in, 6 out]
                    n128 = property on="Bouton Accueil" class="Bool (strict)"("Visible"=FALSE) -> ()  [unwired: 2 in, 2 out]
                    n129 = property on="stop" class="Bool (strict)"("Visible"=TRUE) -> ()  [unwired: 2 in, 2 out]
                    n130 = property on="Start acquisition" class="Bool (strict)"("Visible"=FALSE) -> ()  [unwired: 2 in, 2 out]
                    n131 = Tick Count (ms)() -> (millisecond timer value=w260:u32)
                    n132 = property on="valeur de l'horloge en ms" class="NumNb (strict)"("Value"=w260) -> ()  [unwired: 2 in, 2 out]
                    n133 = property on="Commande onglets" class="Onglet (strict)"("DisabledEnum"=T2."Enabled" ("Désactivé")) -> ()  [unwired: 2 in, 2 out]
                    n134 = property on="Bouton Accueil" class="Bool (strict)"("DisabledEnum"=T2."Disabled and Grayed Out" ("Désactivé")) -> ()  [unwired: 2 in, 2 out]
                  }
                  event "Bouton Accueil": Value Change {
                    w268 = TRUE ("flag")
                    # "Exit"
                    n135 = event-data() -> ()  [unwired: 1 in, 6 out]
                    n136 = Request Deallocation(w268) -> ()
                    n137 = Stop(stop? (T)=w268) -> ()
                  }
                }
              }
            }
            frame Error {
            }
          }
          n138 = property on="Update" class="Ch"("Value"="Press start" ("Étiquette.Texte")) -> ()  [unwired: 2 in, 2 out]
        }
      }
      n139 = property on="Energie UV graph" class="GraphDér (strict)"("History Data"=dbl[] [] ("Données d'historique")) -> ()  [unwired: 2 in, 2 out]
      n140 = property on="Energie UV graph" class="GraphDér (strict)"("Update Mode"=u8 2 ("Mode de rafraîchissement")) -> ()  [unwired: 2 in, 2 out]
      n141 = property on="Puissance depolar graph" class="GraphDér (strict)"("History Data"=dbl[] [] ("Données d'historique")) -> ()  [unwired: 2 in, 2 out]
      n142 = property on="Puissance depolar graph" class="GraphDér (strict)"("Update Mode"=u8 2 ("Mode de rafraîchissement")) -> ()  [unwired: 2 in, 2 out]
      n143 = property on="Energie IR graph" class="GraphDér (strict)"("History Data"=dbl[] [] ("Données d'historique")) -> ()  [unwired: 2 in, 2 out]
      n144 = property on="Energie IR graph" class="GraphDér (strict)"("Update Mode"=u8 2 ("Mode de rafraîchissement")) -> ()  [unwired: 2 in, 2 out]
      n145 = property on="Bouton Accueil" class="Bool (strict)"("Visible"=TRUE) -> ()  [unwired: 2 in, 2 out]
      n146 = property on="Start acquisition" class="Bool (strict)"("Visible"=TRUE) -> ()  [unwired: 2 in, 2 out]
      n147 = property on="stop" class="Bool (strict)"("Visible"=FALSE) -> ()  [unwired: 2 in, 2 out]
      n148 = property on="Bouton Accueil" class="Bool (strict)"("DisabledEnum"=T2."Enabled" ("Désactivé")) -> ()  [unwired: 2 in, 2 out]
      n149 = property on="sortie d'erreur" class="Clust (strict)"("Value"=errorcluster {"status"=FALSE, "code"=0, "source"=""} ("constante d'erreur")) -> ()  [unwired: 2 in, 2 out]
      n150 = property on="Bouton Accueil" class="Bool (strict)"("DisabledEnum"=T2."Enabled" ("Désactivé")) -> ()  [unwired: 2 in, 2 out]
      n151 = property on="Bouton Accueil" class="Bool (strict)"("Value"=FALSE ("Bouton Accueil")) -> ()  [unwired: 2 in, 2 out]
      n152 = property on="Start acquisition" class="Bool (strict)"("Value"=FALSE) -> ()  [unwired: 2 in, 2 out]
      n153 = property on="stop" class="Bool (strict)"("Value"=FALSE ("stop")) -> ()  [unwired: 2 in, 2 out]
      n154 = property on="Scale (Watt or Joule) (Energie UV)" class="MDér (strict)"("DisabledEnum"=T2."Disabled and Grayed Out" ("Désactivé")) -> ()  [unwired: 2 in, 2 out]
      n155 = property on="Scale (Watt or Joule) (Energie UV)" class="MDér (strict)"("DisabledEnum"=T2."Disabled and Grayed Out" ("Désactivé")) -> ()  [unwired: 2 in, 2 out]
      n156 = property on="Scale (Watt or Joule) (Puissance depolar)" class="MDér (strict)"("DisabledEnum"=T2."Disabled and Grayed Out" ("Désactivé")) -> ()  [unwired: 2 in, 2 out]
      n157 = property on="Scale (Watt or Joule) (Puissance depolar)" class="MDér (strict)"("DisabledEnum"=T2."Disabled and Grayed Out" ("Désactivé")) -> ()  [unwired: 2 in, 2 out]
      n158 = property on="Scale (Watt or Joule) (Energie IR)" class="MDér (strict)"("DisabledEnum"=T2."Disabled and Grayed Out" ("Désactivé")) -> ()  [unwired: 2 in, 2 out]
      n159 = property on="Scale (Watt or Joule) (Energie IR)" class="MDér (strict)"("DisabledEnum"=T2."Disabled and Grayed Out" ("Désactivé")) -> ()  [unwired: 2 in, 2 out]
      n160 = property on="Auto Scale (Puissance depolar)" class="Bool (strict)"("Value"=TRUE) -> ()  [unwired: 2 in, 2 out]
      n161 = property on="Auto Scale (Energie UV)" class="Bool (strict)"("Value"=TRUE) -> ()  [unwired: 2 in, 2 out]
      n162 = property on="Auto Scale (Energie IR)" class="Bool (strict)"("Value"=TRUE ("Auto Scale (Energie IR)")) -> ()  [unwired: 2 in, 2 out]
      "Energie IR mean" <- 0.0 ("mean 3")
      "Energie IR variance" <- 0.0 ("rms value 3")
      "Energie IR max" <- 0.0 ("valeur max 3")
      "Energie IR min" <- 0.0 ("valeur min 3")
      "Energie IR value" <- 0.0 ("Numérique 3")
      "Energie IR graph" <- 0.0 ("Graphe déroulant 3")
      "Puissance depolar value" <- 0.0 ("Numérique 2")
      "Puissance depolar graph" <- 0.0 ("Graphe déroulant 2")
      "Puissance depolar mean" <- 0.0 ("mean 2")
      "Puissance depolar variance" <- 0.0 ("rms value 2")
      "Puissance depolar max" <- 0.0 ("valeur max 2")
      "Puissance depolar min" <- 0.0 ("valeur min 2")
      "Energie IR table" <- dbl[] [] ("Tableau 3")
      "Energie IR table (1sec)" <- dbl[] [] ("Tableau1 3")
      "Puissance depolar table" <- dbl[] [] ("Tableau1 2")
      "Energie UV value" <- 0.0 ("Numérique 1")
      "Energie UV graph" <- 0.0 ("Graphe déroulant 1")
      "Energie UV table" <- dbl[] [] ("Tableau 1")
      "Energie UV mean" <- 0.0 ("mean 1")
      "Energie UV variance" <- 0.0 ("rms value 1")
      "Energie UV max" <- 0.0 ("valeur max 1")
      "Energie UV min" <- 0.0 ("valeur min 1")
      "Energie UV table(1sec)" <- dbl[] [] ("Tableau1 1")
      "Taux depolar value" <- 0.0 ("Numérique 7")
      "taux depolar graph" <- 0.0 ("Graphe déroulant 4")
      "Puissance depolar table (stats)" <- dbl[][] [] ("Tableau stat 2")
      "Energie IR table (stats)" <- dbl[][] [] ("Tableau stat 3")
      "Energie UV rapport" <- 0.0 ("rapport 1")
      "Puissance depolar rapport" <- 0.0 ("rapport 2")
      "Energie IR rapport" <- 0.0 ("rapport 3")
      "Taux depolar indicator" <- u32 16777222 ("taux depolar")
      "Puissance depolar table (1sec)" <- dbl[] [] ("Tableau1 2")
      "Energie UV table (stats)" <- dbl[][] [] ("Tableau stat 1")
      "timer 1sec" <- FALSE ("timer 1s")
      "timer 12sec" <- FALSE ("timer 12s")
      "index 1sec" <- 0 ("index 1sec")
      "index 12sec" <- 0 ("index 12sec")
      "Chaîne" <- "Energie UV" ("Chaîne")
      "Chaîne 4" <- "Energie UV (mJ)" ("Chaîne 4")
      "Chaîne 2" <- "Puissance depolar" ("Chaîne 2")
      "Chaîne 3" <- "Energie IR" ("Chaîne 3")
      "Chaîne 5" <- "Energie IR (mJ)" ("Chaîne 5")
      "Chaîne 6" <- "Puissance depolar (W)" ("Chaîne 6")
      "Chaîne 7" <- "Taux depolar" ("Chaîne 7")
      "Update" <- ""
      "chaîne de date/heure" <- ""
      "valeur de l'horloge en ms" <- u32 0 ("valeur de l'horloge en ms")
      "Time" <- ""
      "stop?" <- FALSE ("stop?")
      "Tableau Puissance depolar" <- dbl[] [] ("Tableau Puissance depolar")
      "Tableau UV" <- dbl[] []
      "Tableau IR" <- dbl[] [] ("Tableau IR")
      "taille UV" <- 0.0 ("taille(s)")
      "taille Pd" <- 0.0 ("taille(s) 2")
      "taille IR" <- 0.0 ("taille(s) 3")
      "12sec UV" <- FALSE ("12sec UV")
      "12sec Pd" <- FALSE ("12sec Pd")
      "12sec IR" <- FALSE ("12sec IR")
      "stop UV" <- FALSE ("stop UV")
      "stop Pd" <- FALSE ("stop Pd")
      "stop IR" <- FALSE ("stop IR")
    }
    frame #1 {
      n163 = property on="error IO" class="Clust (strict)"() -> ("Value"=w270:errorcluster)  [unwired: 2 in, 2 out]
      n164 = case shown="Pas d'erreur" w270 {
        selector: w270 -> [_ w1015]
        tunnel: [w274 w1015] -> w269
        frame No Error {
          w282 = T3 {enum."Stop", "Data"=0.0}
          w297 = T3 {enum."Stop", "Data"=0.0}
          w326 = T3 {enum."Stop", "Data"=0.0}
          n165 = property on="Energie UV file (stats)" class="Ref (strict)"() -> ("Value"=w314:refnum<file>)  [unwired: 2 in, 2 out]
          n166 = property on="Puissance depolar file (stats)" class="Ref (strict)"() -> ("Value"=w313:refnum<file>)  [unwired: 2 in, 2 out]
          n167 = property on="Energie IR file (stats)" class="Ref (strict)"() -> ("Value"=w312:refnum<file>)  [unwired: 2 in, 2 out]
          n168 = while {
            tunnel: w314 -> [w700]
            tunnel: w313 -> [w699]
            tunnel: w312 -> [w698]
            stop <- w697 stop-if-true
            # "actions à réaliser toutes les 12sec"
            n169 = event shown="[0] \"12sec\": Valeur changée" {
              selector: _ -> [_ _]
              dyn-events: _ -> [_ _]
              timeout: _ -> [_ _]
              tunnel: w700 -> [w755 _]
              tunnel: w699 -> [w754 _]
              tunnel: w698 -> [w753 _]
              tunnel: [FALSE TRUE] -> w697
              event "12sec": Value Change {
                w747 = ","
                n170 = event-data() -> ()  [unwired: 1 in, 6 out]
                n171 = property on="Tableau UV" class="Tabl (strict)"() -> ("Value"=w721:dbl[])  [unwired: 2 in, 2 out]
                n172 = call <vilib>:"Std Deviation and Variance.vi"("X"=w721) -> ("mean"=w719:dbl, "standard deviation"=w718:dbl)  [unwired: 1 in, 1 out]
                n173 = Array Max & Min(array=w721) -> (max value=w717:dbl, min value=w716:dbl)  [unwired: 2 out]
                n174 = Array Size(array=w721) -> (size(s)=w729:i32)
                n175 = property on="Tableau Puissance depolar" class="Tabl (strict)"() -> ("Value"=w722:dbl[])  [unwired: 2 in, 2 out]
                n176 = To Double Precision Float(number=w729) -> (double precision float=w704:dbl)
                n177 = Get Date/Time In Seconds() -> (seconds since 1Jan1904=w745:timestamp)
                n178 = Format Date/Time String(time format string (%c)="%d-%m-%Y-%H:%M:%S%3u", seconds (now)=w745) -> (date/time string=w748:string)  [unwired: 1 in]
                n179 = Divide(x=w718, y=w719) -> (x/y=w734:dbl)
                n180 = property on="taille UV" class="NumNb (strict)"("Value"=w704) -> ()  [unwired: 2 in, 2 out]
                n181 = property on="Energie UV mean" class="NumNb (strict)"("Value"=w719) -> ()  [unwired: 2 in, 2 out]
                n182 = property on="Energie UV variance" class="NumNb (strict)"("Value"=w718) -> ()  [unwired: 2 in, 2 out]
                n183 = property on="Energie UV max" class="NumNb (strict)"("Value"=w717) -> ()  [unwired: 2 in, 2 out]
                n184 = property on="Energie UV min" class="NumNb (strict)"("Value"=w716) -> ()  [unwired: 2 in, 2 out]
                n185 = Multiply(x=w734, y=100.0) -> (x*y=w715:dbl)
                n186 = property on="valeur de l'horloge en ms" class="NumNb (strict)"() -> ("Value"=w749:u32)  [unwired: 2 in, 2 out]
                n187 = Tick Count (ms)() -> (millisecond timer value=w750:u32)
                n188 = property on="Energie UV rapport" class="NumNb (strict)"("Value"=w715) -> ()  [unwired: 2 in, 2 out]
                n189 = Build Array(w719, w718, w717, w716, w715) -> (w732:dbl[])
                n190 = call <vilib>:"Std Deviation and Variance.vi"("X"=w722) -> ("mean"=w710:dbl, "standard deviation"=w711:dbl)  [unwired: 1 in, 1 out]
                n191 = Array Max & Min(array=w722) -> (max value=w712:dbl, min value=w713:dbl)  [unwired: 2 out]
                n192 = Array Size(array=w722) -> (size(s)=w728:i32)
                n193 = property on="Tableau IR" class="Tabl (strict)"() -> ("Value"=w720:dbl[])  [unwired: 2 in, 2 out]
                n194 = To Double Precision Float(number=w728) -> (double precision float=w703:dbl)
                n195 = Divide(x=w711, y=w710) -> (x/y=w731:dbl)
                n196 = property on="taille Pd" class="NumNb (strict)"("Value"=w703) -> ()  [unwired: 2 in, 2 out]
                n197 = Subtract(x=w750, y=w749) -> (x-y=w751:u32)
                n198 = property on="Puissance depolar mean" class="NumNb (strict)"("Value"=w710) -> ()  [unwired: 2 in, 2 out]
                n199 = property on="Puissance depolar variance" class="NumNb (strict)"("Value"=w711) -> ()  [unwired: 2 in, 2 out]
                n200 = property on="Puissance depolar max" class="NumNb (strict)"("Value"=w712) -> ()  [unwired: 2 in, 2 out]
                n201 = property on="Puissance depolar min" class="NumNb (strict)"("Value"=w713) -> ()  [unwired: 2 in, 2 out]
                n202 = Number To Decimal String(number=w751) -> (decimal integer string=w752:string)  [unwired: 1 in]
                n203 = Multiply(x=w731, y=100.0) -> (x*y=w714:dbl)
                n204 = Build Array(w710, w711, w712, w713, w714) -> (w727:dbl[])
                n205 = Concatenate Strings(w748, w747, w752, w747) -> (w735:string)
                n206 = property on="Puissance depolar rapport" class="NumNb (strict)"("Value"=w714) -> ()  [unwired: 2 in, 2 out]
                n207 = call <vilib>:"Std Deviation and Variance.vi"("X"=w720) -> ("mean"=w705:dbl, "standard deviation"=w706:dbl)  [unwired: 1 in, 1 out]
                n208 = Array Max & Min(array=w720) -> (max value=w707:dbl, min value=w708:dbl)  [unwired: 2 out]
                n209 = Array Size(array=w720) -> (size(s)=w726:i32)
                n210 = To Double Precision Float(number=w726) -> (double precision float=w702:dbl)
                n211 = Divide(x=w706, y=w705) -> (x/y=w724:dbl)
                n212 = property on="taille IR" class="NumNb (strict)"("Value"=w702) -> ()  [unwired: 2 in, 2 out]
                n213 = Multiply(x=w724, y=100.0) -> (x*y=w709:dbl)
                n214 = property on="Energie IR mean" class="NumNb (strict)"("Value"=w705) -> ()  [unwired: 2 in, 2 out]
                n215 = property on="Energie IR variance" class="NumNb (strict)"("Value"=w706) -> ()  [unwired: 2 in, 2 out]
                n216 = property on="Energie IR max" class="NumNb (strict)"("Value"=w707) -> ()  [unwired: 2 in, 2 out]
                n217 = property on="Energie IR min" class="NumNb (strict)"("Value"=w708) -> ()  [unwired: 2 in, 2 out]
                n218 = Build Array(w705, w706, w707, w708, w709) -> (w723:dbl[])
                n219 = property on="Energie IR rapport" class="NumNb (strict)"("Value"=w709) -> ()  [unwired: 2 in, 2 out]
                n220 = Array To Spreadsheet String(array=w732, 3:"%f" ("chaîne de format")) -> (spreadsheet string=w743:string)  [unwired: 1 in]
                n221 = Array To Spreadsheet String(array=w727, 3:"%f" ("chaîne de format")) -> (spreadsheet string=w740:string)  [unwired: 1 in]
                n222 = Array To Spreadsheet String(array=w723, 3:"%f" ("chaîne de format")) -> (spreadsheet string=w737:string)  [unwired: 1 in]
                n223 = Concatenate Strings(w735, w743) -> (w742:string)
                n224 = Concatenate Strings(w735, w740) -> (w739:string)
                n225 = Concatenate Strings(w735, w737) -> (w736:string)
                n226 = Write to Text File(file (use dialog)=w755, text=w742) -> ()  [unwired: 2 in, 3 out]
                n227 = Write to Text File(file (use dialog)=w754, text=w739) -> ()  [unwired: 2 in, 3 out]
                n228 = Write to Text File(file (use dialog)=w753, text=w736) -> ()  [unwired: 2 in, 3 out]
              }
              event "stop": Value Change {
                n229 = event-data() -> ()  [unwired: 1 in, 6 out]
                n230 = property on="stop UV" class="Bool (strict)"("Val(Sgnl)"=TRUE ("Valeur (Signalisation)")) -> ()  [unwired: 2 in, 2 out]
                n231 = property on="stop Pd" class="Bool (strict)"("Val(Sgnl)"=TRUE ("Valeur (Signalisation)")) -> ()  [unwired: 2 in, 2 out]
                n232 = property on="stop IR" class="Bool (strict)"("Val(Sgnl)"=TRUE ("Valeur (Signalisation)")) -> ()  [unwired: 2 in, 2 out]
              }
            }
          }
          n233 = Obtain Queue(name (unnamed)="Energie UV" ("nom (aucun)"), element data type=w326) -> (queue out=w327:refnum<queue>, error out=w328:errorcluster)  [unwired: 3 in, 1 out]
          n234 = property on="COM Port table" class="Tabl (strict)"() -> ("Value"=w320:refnum<visa-resource-name>[])  [unwired: 2 in, 2 out]
          n235 = Bundle(cluster=w326, enum16{"Init", "Read", "Stop", "12sec"}."Init") -> (w329:T3)  [unwired: 1 in]
          n236 = Enqueue Element At Opposite End(queue=w327, element=w329, error in (no error)=w328) -> (queue out=w325:refnum<queue>, error out=w308:errorcluster)  [unwired: 1 in, 1 out]
          n237 = Index Array(array=w320, index=0 ("indice")) -> (element=w272:refnum<visa-resource-name>)
          n238 = while {
            shift-right: [w831] -> w324
            shift-left: w308 -> [w838]
            shift-right: [w830] -> w323
            shift-left: w325 -> [w832]
            shift-right: [w827] -> _
            shift-left: _ -> [w828]
            stop <- w829 stop-if-true
            n239 = Dequeue Element(queue=w832, error in (no error)=w838) -> (queue out=w833:refnum<queue>, element=w837:T3, error out=w834:errorcluster)  [unwired: 1 in, 1 out]
            n240 = Unbundle(w837) -> (w836:enum16{"Init", "Read", "Stop", "12sec"}, "Data"=w835:dbl)
            n241 = case shown="\"Read\"" w836 {
              tunnel: w828 -> [_ w844 w851 w863]
              tunnel: w835 -> [_ w843 w852 _]
              tunnel: w834 -> [w842 w848 w857 w868]
              tunnel: w833 -> [w840 w846 w855 w867]
              tunnel: [w842 w848 w857 w866] -> w831
              tunnel: [FALSE FALSE FALSE TRUE] -> w829
              tunnel: [w840 w846 w855 w864] -> w830
              tunnel: [dbl[] [] w845 dbl[] [] w863] -> w827
              frame "Init", Default {
              }
              frame "Read" {
                n242 = Insert Into Array(array=w844, new element=w843) -> (w845:dbl[])  [unwired: 1 in]
                n243 = property on="Tableau UV" class="Tabl (strict)"("Value"=w845) -> ()  [unwired: 2 in, 2 out]
              }
              frame "12sec" {
                n244 = Equal To 0?(x=w852) -> (x = 0?=w853:bool)
                n245 = case shown="Vrai" w853 {
                  tunnel: w852 -> [w858 _]
                  tunnel: w851 -> [_ w859]
                  tunnel: [w858 w862] -> w850
                  frame False {
                  }
                  frame True {
                    n246 = Array Size(array=w859) -> (size(s)=w861:i32)
                    n247 = Decrement(x=w861) -> (x-1=w860:i32)
                    n248 = Index Array(array=w859, index=w860) -> (element=w862:dbl)
                  }
                }
                n249 = Insert Into Array(array=w851, new element=w850) -> (w854:dbl[])  [unwired: 1 in]
                n250 = property on="Tableau UV" class="Tabl (strict)"("Value"=w854) -> ()  [unwired: 2 in, 2 out]
              }
              frame "Stop" {
                n251 = Flush Queue(queue=w867, error in (no error)=w868) -> (queue out=w864:refnum<queue>, error out=w866:errorcluster)  [unwired: 1 out]
              }
            }
          }
          n252 = while {
            tunnel: w326 -> [w878]
            shift-right: [w877] -> w310
            shift-left: w308 -> [w876]
            shift-right: [w875] -> _
            shift-left: w325 -> [w879]
            shift-right: [w871] -> w309
            shift-left: w308 -> [w872]
            shift-right: [w869] -> _
            shift-left: w272 -> [w873]
            stop <- w874 stop-if-true
            n253 = event shown="[0] Timeout" {
              selector: _ -> [_ _ _ _ _ _ _ _ _]
              dyn-events: _ -> [_ _ _ _ _ _ _ _ _]
              timeout: 1 -> [_ _ _ _ _ _ _ _ _]
              tunnel: w879 -> [w895 w912 w922 w937 w960 w973 w986 w999 w1012]
              tunnel: w878 -> [w894 w911 w925 _ _ _ _ _ _]
              tunnel: [w890 w907 w920 w936 w959 w972 w985 w998 w1011] -> w877
              tunnel: w876 -> [w892 w909 w923 w936 w959 w972 w985 w998 w1011]
              tunnel: [w891 w908 w924 w937 w960 w973 w986 w999 w1012] -> w875
              tunnel: [w889 w906 w919 FALSE w957 w969 w982 w995 w1008] -> w874
              tunnel: w873 -> [w880 w900 w915 w931 w954 w965 w978 w991 w1004]
              tunnel: w872 -> [w881 w899 w914 w932 w953 w966 w979 w992 w1005]
              tunnel: [w884 w898 w914 w927 w952 w964 w977 w990 w1003] -> w871
              tunnel: [w883 w897 w915 w929 w951 w963 w976 w989 w1002] -> w869
              event Timeout {
                n254 = event-data() -> ()  [unwired: 1 in, 1 out]
                n255 = call "Read Single Value (SubVI).vi"("entrée d'erreur (pas d'erreur)"=w881, "Refnum VISA en entrée"=w880) -> ("sortie d'erreur"=w884:errorcluster, "nombre"=w885:dbl, "Refnum VISA en sortie"=w883:refnum<visa-resource-name>)  [unwired: 6 in, 1 out]
                n256 = Bundle(cluster=w894, enum16{"Init", "Read", "Stop", "12sec"}."Read", "Data"=w885) -> (w893:T3)
                n257 = Enqueue Element(queue=w895, element=w893, error in (no error)=w892) -> (queue out=w891:refnum<queue>, error out=w890:errorcluster)  [unwired: 1 in, 1 out]
                n258 = Unbundle By Name(w890) -> ("status"=w887:bool)
                n259 = Unbundle By Name(w884) -> ("status"=w886:bool)
                n260 = Compound Arithmetic op=OR ("Opérateur arithmétique")(w886, w887, FALSE) -> (w889:bool)
              }
              event "12sec UV": Value Change {
                n261 = event-data() -> ()  [unwired: 1 in, 1 out]
                n262 = call "Read Single Value (SubVI).vi"("entrée d'erreur (pas d'erreur)"=w899, "Refnum VISA en entrée"=w900) -> ("sortie d'erreur"=w898:errorcluster, "nombre"=w896:dbl, "Refnum VISA en sortie"=w897:refnum<visa-resource-name>)  [unwired: 6 in, 1 out]
                n263 = Bundle(cluster=w911, enum16{"Init", "Read", "Stop", "12sec"}."12sec", "Data"=w896) -> (w910:T3)
                n264 = Enqueue Element(queue=w912, element=w910, error in (no error)=w909) -> (queue out=w908:refnum<queue>, error out=w907:errorcluster)  [unwired: 1 in, 1 out]
                n265 = Unbundle By Name(w907) -> ("status"=w904:bool)
                n266 = Unbundle By Name(w898) -> ("status"=w903:bool)
                n267 = property on="12sec UV" class="Bool (strict)"("Value"=FALSE ("12sec UV")) -> ()  [unwired: 2 in, 2 out]
                n268 = Compound Arithmetic op=OR ("Opérateur arithmétique")(w903, w904, FALSE) -> (w906:bool)
              }
              event "stop UV": Value Change {
                n269 = event-data() -> ()  [unwired: 1 in, 6 out]
                n270 = Bundle(cluster=w925, enum16{"Init", "Read", "Stop", "12sec"}."Stop") -> (w921:T3)  [unwired: 1 in]
                n271 = Enqueue Element(queue=w922, element=w921, error in (no error)=w923) -> (queue out=w924:refnum<queue>, error out=w920:errorcluster)  [unwired: 1 in, 1 out]
                n272 = Unbundle By Name(w920) -> ("status"=w917:bool)
                n273 = Unbundle By Name(w914) -> ("status"=w916:bool)
                n274 = Compound Arithmetic op=OR ("Opérateur arithmétique")(w916, w917, TRUE) -> (w919:bool)
              }
              event "Auto Scale (Energie UV)": Value Change {
                w926 = u32 100
                n275 = event-data() -> ("NewVal"=w934:bool)  [unwired: 1 in, 5 out]
                n276 = call "Wait (SubVI).vi"("error in"=w932, "attente (ms)"=w926) -> ("error out"=w928:errorcluster)  [unwired: 25 in]
                n277 = case shown="Faux" w934 {
                  tunnel: [T2."Enabled" ("Désactivé") T2."Disabled and Grayed Out" ("Désactivé")] -> w933
                  tunnel: w931 -> [w939 w945]
                  tunnel: [w942 w946] -> w929
                  tunnel: w928 -> [w941 w948]
                  tunnel: [w940 w947] -> w930
                  frame False {
                    n278 = call "Port Write (SubVI).vi"("error in"=w941, "write buffer"="*SAS0", "VISA Refnum in"=w939) -> ("error out"=w940:errorcluster, "VISA Refnum out"=w942:refnum<visa-resource-name>)  [unwired: 1 in]
                  }
                  frame True {
                    n279 = call "Port Write (SubVI).vi"("error in"=w948, "write buffer"="*SAS1", "VISA Refnum in"=w945) -> ("error out"=w947:errorcluster, "VISA Refnum out"=w946:refnum<visa-resource-name>)  [unwired: 1 in]
                  }
                }
                n280 = property on="Scale (Watt or Joule) (Energie UV)" class="MDér (strict)"("DisabledEnum"=w933) -> ()  [unwired: 2 in, 2 out]
                n281 = call "Wait (SubVI).vi"("error in"=w930, "attente (ms)"=w926) -> ("error out"=w927:errorcluster)  [unwired: 25 in]
              }
              event "Scale (Watt or Joule) (Energie UV)": Value Change {
                w950 = u32 100 ("attente (ms)")
                n282 = event-data() -> ()  [unwired: 1 in, 6 out]
                n283 = property on="Scale (Watt or Joule) (Energie UV)" class="MDér (strict)"() -> ("Value"=w962:i32)  [unwired: 2 in, 2 out]
                n284 = call "Wait (SubVI).vi"("error in"=w953, "attente (ms)"=w950) -> ("error out"=w958:errorcluster)  [unwired: 25 in]
                n285 = call "Set Scale (SubVI).vi"("error in"=w958, "Scale"=w962, "VISA Refnum in"=w954) -> ("error out"=w961:errorcluster, "VISA Refnum out"=w951:refnum<visa-resource-name>)
                n286 = call "Wait (SubVI).vi"("error in"=w961, "attente (ms)"=w950) -> ("error out"=w952:errorcluster)  [unwired: 25 in]
                n287 = Unbundle By Name(w952) -> ("status"=w956:bool)
                n288 = Compound Arithmetic op=OR ("Opérateur arithmétique")(w956, FALSE) -> (w957:bool)
              }
              event "Trigger Level (% of Scale) (Energie UV)": Value Change {
                w970 = u32 100 ("milliseconds to wait")
                n289 = event-data() -> ()  [unwired: 1 in, 6 out]
                n290 = property on="Trigger Level (% of Scale) (Energie UV)" class="NumNb (strict)"() -> ("Value"=w974:dbl)  [unwired: 2 in, 2 out]
                n291 = call "Wait (SubVI).vi"("error in"=w966, "attente (ms)"=w970) -> ("error out"=w971:errorcluster)  [unwired: 25 in]
                n292 = call "Set Trigger Level (SubVI).vi"("error in"=w971, "Trigger Level (% of Scale)"=w974, "VISA Refnum in"=w965) -> ("error out"=w975:errorcluster, "VISA Refnum out"=w963:refnum<visa-resource-name>)
                n293 = call "Wait (SubVI).vi"("error in"=w975, "attente (ms)"=w970) -> ("error out"=w964:errorcluster)  [unwired: 25 in]
                n294 = Unbundle By Name(w964) -> ("status"=w968:bool)
                n295 = Compound Arithmetic op=OR ("Opérateur arithmétique")(w968, FALSE) -> (w969:bool)
              }
              event "Multiplier (Energie UV)": Value Change {
                w983 = u32 100 ("milliseconds to wait")
                n296 = event-data() -> ()  [unwired: 1 in, 6 out]
                n297 = call "Wait (SubVI).vi"("error in"=w979, "attente (ms)"=w983) -> ("error out"=w984:errorcluster)  [unwired: 25 in]
                n298 = property on="Multiplier (Energie UV)" class="NumNb (strict)"() -> ("Value"=w987:sgl)  [unwired: 2 in, 2 out]
                n299 = call "Set Multiplier (SubVI).vi"("error in"=w984, "Multiplier"=w987, "VISA Refnum in"=w978) -> ("error out"=w988:errorcluster, "VISA Refnum out"=w976:refnum<visa-resource-name>)
                n300 = call "Wait (SubVI).vi"("error in"=w988, "attente (ms)"=w983) -> ("error out"=w977:errorcluster)  [unwired: 25 in]
                n301 = Unbundle By Name(w977) -> ("status"=w980:bool)
                n302 = Compound Arithmetic op=OR ("Opérateur arithmétique")(w980, FALSE) -> (w982:bool)
              }
              event "Offset (Energie UV)": Value Change {
                w996 = u32 100 ("milliseconds to wait")
                n303 = event-data() -> ()  [unwired: 1 in, 6 out]
                n304 = call "Wait (SubVI).vi"("error in"=w992, "attente (ms)"=w996) -> ("error out"=w997:errorcluster)  [unwired: 25 in]
                n305 = property on="Offset (Energie UV)" class="NumNb (strict)"() -> ("Value"=w1000:sgl)  [unwired: 2 in, 2 out]
                n306 = call "Set Offset (SubVI).vi"("error in"=w997, "Offset in"=w1000, "VISA Refnum in"=w991) -> ("error out"=w1001:errorcluster, "VISA Refnum out"=w989:refnum<visa-resource-name>)
                n307 = call "Wait (SubVI).vi"("error in"=w1001, "attente (ms)"=w996) -> ("error out"=w990:errorcluster)  [unwired: 25 in]
                n308 = Unbundle By Name(w990) -> ("status"=w993:bool)
                n309 = Compound Arithmetic op=OR ("Opérateur arithmétique")(w993, FALSE) -> (w995:bool)
              }
              event "Wavelength (nm) (Energie UV)": Value Change {
                w1009 = u32 100 ("milliseconds to wait")
                n310 = event-data() -> ()  [unwired: 1 in, 6 out]
                n311 = property on="Wavelength (nm) (Energie UV)" class="NumNb (strict)"() -> ("Value"=w1013:u32)  [unwired: 2 in, 2 out]
                n312 = call "Wait (SubVI).vi"("error in"=w1005, "attente (ms)"=w1009) -> ("error out"=w1010:errorcluster)  [unwired: 25 in]
                n313 = call "Set Wavelength (SubVI).vi"("error in"=w1010, "Wavelength (nm)"=w1013, "VISA Refnum in"=w1004) -> ("error out"=w1014:errorcluster, "VISA Refnum out"=w1002:refnum<visa-resource-name>)
                n314 = call "Wait (SubVI).vi"("error in"=w1014, "attente (ms)"=w1009) -> ("error out"=w1003:errorcluster)  [unwired: 25 in]
                n315 = Unbundle By Name(w1003) -> ("status"=w1006:bool)
                n316 = Compound Arithmetic op=OR ("Opérateur arithmétique")(w1006, FALSE) -> (w1008:bool)
              }
            }
          }
          n317 = Release Queue(queue=w323, error in (no error)=w324) -> (error out=w311:errorcluster)  [unwired: 1 in, 2 out]
          n318 = Merge Errors(w309, w310, w311) -> (w275:errorcluster)
          n319 = Obtain Queue(name (unnamed)="Puissance depolar" ("nom (aucun)"), element data type=w297) -> (queue out=w296:refnum<queue>, error out=w295:errorcluster)  [unwired: 3 in, 1 out]
          n320 = while {
            shift-right: [w763] -> _
            shift-left: 0.0 -> [w762]
            stop <- w765 stop-if-true
            n321 = Equal?(x=w762, y=11.0) -> (x = y?=w761:bool)
            n322 = case shown="Vrai" w761 {
              selector: w761 -> [w769 _]
              tunnel: [0.0 w772] -> w763
              tunnel: w762 -> [_ w771]
              frame True {
                n323 = property on="12sec" class="Bool (strict)"("Val(Sgnl)"=w769) -> ()  [unwired: 2 in, 2 out]
                n324 = property on="12sec UV" class="Bool (strict)"("Val(Sgnl)"=TRUE ("12sec UV")) -> ()  [unwired: 2 in, 2 out]
                n325 = property on="12sec Pd" class="Bool (strict)"("Val(Sgnl)"=TRUE ("12sec Pd")) -> ()  [unwired: 2 in, 2 out]
                n326 = property on="12sec IR" class="Bool (strict)"("Val(Sgnl)"=TRUE ("12sec IR")) -> ()  [unwired: 2 in, 2 out]
              }
              frame False {
                n327 = Increment(x=w771) -> (x+1=w772:dbl)
              }
            }
            n328 = Wait (ms)(milliseconds to wait=u32 1000 ("attente (ms)")) -> ()  [unwired: 1 out]
            n329 = property on="stop" class="Bool (strict)"() -> ("Value"=w765:bool)  [unwired: 2 in, 2 out]
          }
          n330 = property on="COM Port table" class="Tabl (strict)"() -> ("Value"=w302:refnum<visa-resource-name>[])  [unwired: 2 in, 2 out]
          n331 = Bundle(cluster=w297, enum16{"Init", "Read", "Stop", "12sec"}."Init") -> (w294:T3)  [unwired: 1 in]
          n332 = Enqueue Element At Opposite End(queue=w296, element=w294, error in (no error)=w295) -> (queue out=w298:refnum<queue>, error out=w307:errorcluster)  [unwired: 1 in, 1 out]
          n333 = Index Array(array=w302, index=1 ("indice")) -> (element=w273:refnum<visa-resource-name>)
          n334 = while {
            shift-right: [w516] -> w299
            shift-left: w307 -> [w523]
            shift-right: [w515] -> w300
            shift-left: w298 -> [w517]
            shift-right: [w512] -> _
            shift-left: _ -> [w513]
            stop <- w514 stop-if-true
            n335 = Dequeue Element(queue=w517, error in (no error)=w523) -> (queue out=w518:refnum<queue>, element=w522:T3, error out=w519:errorcluster)  [unwired: 1 in, 1 out]
            n336 = Unbundle(w522) -> (w521:enum16{"Init", "Read", "Stop", "12sec"}, "Data"=w520:dbl)
            n337 = case shown="\"Read\"" w521 {
              tunnel: w513 -> [_ w530 w537 w541]
              tunnel: w520 -> [_ w529 w536 _]
              tunnel: w519 -> [w527 w534 w540 w546]
              tunnel: w518 -> [w525 w532 w538 w545]
              tunnel: [w527 w534 w540 w544] -> w516
              tunnel: [FALSE FALSE FALSE TRUE] -> w514
              tunnel: [w525 w532 w538 w542] -> w515
              tunnel: [dbl[] [] dbl[] [] w535 w541] -> w512
              frame "Init", Default {
              }
              frame "12sec" {
                n338 = Insert Into Array(array=w530, new element=w529) -> (w531:dbl[])  [unwired: 1 in]
                n339 = property on="Tableau Puissance depolar" class="Tabl (strict)"("Value"=w531) -> ()  [unwired: 2 in, 2 out]
              }
              frame "Read" {
                n340 = Insert Into Array(array=w537, new element=w536) -> (w535:dbl[])  [unwired: 1 in]
                n341 = property on="Tableau Puissance depolar" class="Tabl (strict)"("Value"=w535) -> ()  [unwired: 2 in, 2 out]
              }
              frame "Stop" {
                n342 = Flush Queue(queue=w545, error in (no error)=w546) -> (queue out=w542:refnum<queue>, error out=w544:errorcluster)  [unwired: 1 out]
              }
            }
          }
          n343 = while {
            tunnel: w297 -> [w556]
            shift-right: [w555] -> w305
            shift-left: w307 -> [w554]
            shift-right: [w553] -> _
            shift-left: w298 -> [w557]
            shift-right: [w549] -> w306
            shift-left: w307 -> [w550]
            shift-right: [w547] -> _
            shift-left: w273 -> [w551]
            stop <- w552 stop-if-true
            n344 = event shown="[0] Timeout" {
              selector: _ -> [_ _ _ _ _ _ _ _ _]
              dyn-events: _ -> [_ _ _ _ _ _ _ _ _]
              timeout: 100 -> [_ _ _ _ _ _ _ _ _]
              tunnel: w557 -> [w575 w594 w604 w619 w642 w655 w668 w681 w694]
              tunnel: w556 -> [w574 w593 w607 _ _ _ _ _ _]
              tunnel: [w570 w589 w602 w618 w641 w654 w667 w680 w693] -> w555
              tunnel: w554 -> [w572 w591 w605 w618 w641 w654 w667 w680 w693]
              tunnel: [w571 w590 w606 w619 w642 w655 w668 w681 w694] -> w553
              tunnel: [w569 w588 w601 FALSE w639 w651 w664 w677 w690] -> w552
              tunnel: w551 -> [w559 w577 w597 w614 w633 w646 w660 w672 w685]
              tunnel: w550 -> [w562 w580 w595 w612 w636 w648 w661 w674 w687]
              tunnel: [w561 w579 w595 w609 w635 w647 w659 w673 w686] -> w549
              tunnel: [w560 w578 w597 w613 w632 w645 w658 w671 w684] -> w547
              event Timeout {
                n345 = event-data() -> ()  [unwired: 1 in, 3 out]
                n346 = call "Read Single Value (SubVI).vi"("entrée d'erreur (pas d'erreur)"=w562, "Refnum VISA en entrée"=w559) -> ("sortie d'erreur"=w561:errorcluster, "nombre"=w558:dbl, "Refnum VISA en sortie"=w560:refnum<visa-resource-name>)  [unwired: 6 in, 1 out]
                n347 = Divide(x=w558, y=1000.0) -> (x/y=w564:dbl)
                n348 = Bundle(cluster=w574, enum16{"Init", "Read", "Stop", "12sec"}."Read", "Data"=w564) -> (w573:T3)
                n349 = Enqueue Element(queue=w575, element=w573, error in (no error)=w572) -> (queue out=w571:refnum<queue>, error out=w570:errorcluster)  [unwired: 1 in, 1 out]
                n350 = Unbundle By Name(w570) -> ("status"=w567:bool)
                n351 = Unbundle By Name(w561) -> ("status"=w566:bool)
                n352 = Compound Arithmetic op=OR ("Opérateur arithmétique")(w566, w567, FALSE) -> (w569:bool)
              }
              event "12sec Pd": Value Change {
                n353 = event-data() -> ()  [unwired: 1 in, 1 out]
                n354 = call "Read Single Value (SubVI).vi"("entrée d'erreur (pas d'erreur)"=w580, "Refnum VISA en entrée"=w577) -> ("sortie d'erreur"=w579:errorcluster, "nombre"=w576:dbl, "Refnum VISA en sortie"=w578:refnum<visa-resource-name>)  [unwired: 6 in, 1 out]
                n355 = Divide(x=w576, y=1000.0) -> (x/y=w583:dbl)
                n356 = Bundle(cluster=w593, enum16{"Init", "Read", "Stop", "12sec"}."12sec", "Data"=w583) -> (w592:T3)
                n357 = property on="12sec Pd" class="Bool (strict)"("Value"=FALSE ("12sec Pd")) -> ()  [unwired: 2 in, 2 out]
                n358 = Enqueue Element(queue=w594, element=w592, error in (no error)=w591) -> (queue out=w590:refnum<queue>, error out=w589:errorcluster)  [unwired: 1 in, 1 out]
                n359 = Unbundle By Name(w589) -> ("status"=w586:bool)
                n360 = Unbundle By Name(w579) -> ("status"=w585:bool)
                n361 = Compound Arithmetic op=OR ("Opérateur arithmétique")(w585, w586, FALSE) -> (w588:bool)
              }
              event "stop Pd": Value Change {
                n362 = event-data() -> ()  [unwired: 1 in, 6 out]
                n363 = Bundle(cluster=w607, enum16{"Init", "Read", "Stop", "12sec"}."Stop") -> (w603:T3)  [unwired: 1 in]
                n364 = Enqueue Element(queue=w604, element=w603, error in (no error)=w605) -> (queue out=w606:refnum<queue>, error out=w602:errorcluster)  [unwired: 1 in, 1 out]
                n365 = Unbundle By Name(w602) -> ("status"=w599:bool)
                n366 = Unbundle By Name(w595) -> ("status"=w598:bool)
                n367 = Compound Arithmetic op=OR ("Opérateur arithmétique")(w598, w599, TRUE) -> (w601:bool)
              }
              event "Auto Scale (Energie UV)": Value Change {
                w608 = u32 100
                n368 = event-data() -> ("NewVal"=w616:bool)  [unwired: 1 in]
                n369 = call "Wait (SubVI).vi"("error in"=w612, "attente (ms)"=w608) -> ("error out"=w610:errorcluster)  [unwired: 25 in]
                n370 = case shown="Vrai" w616 {
                  tunnel: [T2."Enabled" ("Désactivé") T2."Disabled and Grayed Out" ("Désactivé")] -> w615
                  tunnel: w614 -> [w621 w627]
                  tunnel: [w624 w628] -> w613
                  tunnel: w610 -> [w623 w630]
                  tunnel: [w622 w629] -> w611
                  frame False {
                    n371 = call "Port Write (SubVI).vi"("error in"=w623, "write buffer"="*SAS0", "VISA Refnum in"=w621) -> ("error out"=w622:errorcluster, "VISA Refnum out"=w624:refnum<visa-resource-name>)  [unwired: 1 in]
                  }
                  frame True {
                    n372 = call "Port Write (SubVI).vi"("error in"=w630, "write buffer"="*SAS1", "VISA Refnum in"=w627) -> ("error out"=w629:errorcluster, "VISA Refnum out"=w628:refnum<visa-resource-name>)  [unwired: 1 in]
                  }
                }
                n373 = property on="Scale (Watt or Joule) (Puissance depolar)" class="MDér (strict)"("DisabledEnum"=w615) -> ()  [unwired: 2 in, 2 out]
                n374 = call "Wait (SubVI).vi"("error in"=w611, "attente (ms)"=w608) -> ("error out"=w609:errorcluster)  [unwired: 25 in]
              }
              event "Scale (Watt or Joule) (Energie UV)": Value Change {
                w634 = u32 100 ("attente (ms)")
                n375 = event-data() -> ()  [unwired: 1 in, 6 out]
                n376 = property on="Scale (Watt or Joule) (Puissance depolar)" class="MDér (strict)"() -> ("Value"=w644:u16)  [unwired: 2 in, 2 out]
                n377 = call "Wait (SubVI).vi"("error in"=w636, "attente (ms)"=w634) -> ("error out"=w640:errorcluster)  [unwired: 25 in]
                n378 = call "Set Scale (SubVI).vi"("error in"=w640, "Scale"=w644, "VISA Refnum in"=w633) -> ("error out"=w643:errorcluster, "VISA Refnum out"=w632:refnum<visa-resource-name>)
                n379 = call "Wait (SubVI).vi"("error in"=w643, "attente (ms)"=w634) -> ("error out"=w635:errorcluster)  [unwired: 25 in]
                n380 = Unbundle By Name(w635) -> ("status"=w638:bool)
                n381 = Compound Arithmetic op=OR ("Opérateur arithmétique")(w638, FALSE) -> (w639:bool)
              }
              event "Trigger Level (% of Scale) (Energie UV)": Value Change {
                w652 = u32 100 ("milliseconds to wait")
                n382 = event-data() -> ()  [unwired: 1 in, 6 out]
                n383 = property on="Trigger Level (% of Scale) (Puissance depolar)" class="NumNb (strict)"() -> ("Value"=w656:dbl)  [unwired: 2 in, 2 out]
                n384 = call "Wait (SubVI).vi"("error in"=w648, "attente (ms)"=w652) -> ("error out"=w653:errorcluster)  [unwired: 25 in]
                n385 = call "Set Trigger Level (SubVI).vi"("error in"=w653, "Trigger Level (% of Scale)"=w656, "VISA Refnum in"=w646) -> ("error out"=w657:errorcluster, "VISA Refnum out"=w645:refnum<visa-resource-name>)
                n386 = call "Wait (SubVI).vi"("error in"=w657, "attente (ms)"=w652) -> ("error out"=w647:errorcluster)  [unwired: 25 in]
                n387 = Unbundle By Name(w647) -> ("status"=w650:bool)
                n388 = Compound Arithmetic op=OR ("Opérateur arithmétique")(w650, FALSE) -> (w651:bool)
              }
              event "Multiplier (Energie UV)": Value Change {
                w665 = u32 100 ("milliseconds to wait")
                n389 = event-data() -> ()  [unwired: 1 in, 6 out]
                n390 = call "Wait (SubVI).vi"("error in"=w661, "attente (ms)"=w665) -> ("error out"=w666:errorcluster)  [unwired: 25 in]
                n391 = property on="Multiplier (Puissance depolar)" class="NumNb (strict)"() -> ("Value"=w669:sgl)  [unwired: 2 in, 2 out]
                n392 = call "Set Multiplier (SubVI).vi"("error in"=w666, "Multiplier"=w669, "VISA Refnum in"=w660) -> ("error out"=w670:errorcluster, "VISA Refnum out"=w658:refnum<visa-resource-name>)
                n393 = call "Wait (SubVI).vi"("error in"=w670, "attente (ms)"=w665) -> ("error out"=w659:errorcluster)  [unwired: 25 in]
                n394 = Unbundle By Name(w659) -> ("status"=w662:bool)
                n395 = Compound Arithmetic op=OR ("Opérateur arithmétique")(w662, FALSE) -> (w664:bool)
              }
              event "Offset (Energie UV)": Value Change {
                w678 = u32 100 ("milliseconds to wait")
                n396 = event-data() -> ()  [unwired: 1 in, 6 out]
                n397 = call "Wait (SubVI).vi"("error in"=w674, "attente (ms)"=w678) -> ("error out"=w679:errorcluster)  [unwired: 25 in]
                n398 = property on="Offset (Puissance depolar)" class="NumNb (strict)"() -> ("Value"=w682:sgl)  [unwired: 2 in, 2 out]
                n399 = call "Set Offset (SubVI).vi"("error in"=w679, "Offset in"=w682, "VISA Refnum in"=w672) -> ("error out"=w683:errorcluster, "VISA Refnum out"=w671:refnum<visa-resource-name>)
                n400 = call "Wait (SubVI).vi"("error in"=w683, "attente (ms)"=w678) -> ("error out"=w673:errorcluster)  [unwired: 25 in]
                n401 = Unbundle By Name(w673) -> ("status"=w675:bool)
                n402 = Compound Arithmetic op=OR ("Opérateur arithmétique")(w675, FALSE) -> (w677:bool)
              }
              event "Wavelength (nm) (Energie UV)": Value Change {
                w691 = u32 100 ("milliseconds to wait")
                n403 = event-data() -> ()  [unwired: 1 in, 6 out]
                n404 = property on="Wavelength (nm) (Puissance depolar)" class="NumNb (strict)"() -> ("Value"=w695:u32)  [unwired: 2 in, 2 out]
                n405 = call "Wait (SubVI).vi"("error in"=w687, "attente (ms)"=w691) -> ("error out"=w692:errorcluster)  [unwired: 25 in]
                n406 = call "Set Wavelength (SubVI).vi"("error in"=w692, "Wavelength (nm)"=w695, "VISA Refnum in"=w685) -> ("error out"=w696:errorcluster, "VISA Refnum out"=w684:refnum<visa-resource-name>)
                n407 = call "Wait (SubVI).vi"("error in"=w696, "attente (ms)"=w691) -> ("error out"=w686:errorcluster)  [unwired: 25 in]
                n408 = Unbundle By Name(w686) -> ("status"=w688:bool)
                n409 = Compound Arithmetic op=OR ("Opérateur arithmétique")(w688, FALSE) -> (w690:bool)
              }
            }
          }
          n410 = property on="Update" class="Ch"("Value"="Data acquisition" ("Étiquette.Texte")) -> ()  [unwired: 2 in, 2 out]
          n411 = property on="Energie UV file (1sec)" class="Ref (strict)"() -> ("Value"=w317:refnum<file>)  [unwired: 2 in, 2 out]
          n412 = property on="Puissance depolar file (1sec)" class="Ref (strict)"() -> ("Value"=w319:refnum<file>)  [unwired: 2 in, 2 out]
          n413 = property on="Energie IR file (1sec)" class="Ref (strict)"() -> ("Value"=w318:refnum<file>)  [unwired: 2 in, 2 out]
          n414 = while {
            tunnel: w319 -> [w800]
            tunnel: w318 -> [w789]
            tunnel: w317 -> [w788]
            stop <- w823 stop-if-true
            w796 = ","
            w797 = "\r\n"
            # "actions à réaliser toutes les 1sec"
            n415 = property on="Tableau Puissance depolar" class="Tabl (strict)"() -> ("Value"=w784:dbl[])  [unwired: 2 in, 2 out]
            n416 = property on="Tableau IR" class="Tabl (strict)"() -> ("Value"=w779:dbl[])  [unwired: 2 in, 2 out]
            n417 = property on="Tableau UV" class="Tabl (strict)"() -> ("Value"=w781:dbl[])  [unwired: 2 in, 2 out]
            n418 = Array Size(array=w781) -> (size(s)=w778:i32)
            n419 = Array Size(array=w784) -> (size(s)=w776:i32)
            n420 = Subtract(x=w778, y=10) -> (x-y=w787:i32)
            n421 = Array Size(array=w779) -> (size(s)=w774:i32)
            n422 = Subtract(x=w776, y=1) -> (x-y=w786:i32)
            n423 = Subtract(x=w774, y=10) -> (x-y=w785:i32)
            n424 = Index Array(array=w781, index=w787) -> (element=w780:dbl)
            n425 = Get Date/Time In Seconds() -> (seconds since 1Jan1904=w799:timestamp)
            n426 = Format Date/Time String(time format string (%c)="%d-%m-%Y-%H:%M:%S%3u", seconds (now)=w799) -> (date/time string=w795:string)  [unwired: 1 in]
            n427 = Index Array(array=w784, index=w786) -> (element=w782:dbl)
            n428 = Index Array(array=w779, index=w785) -> (element=w783:dbl)
            n429 = property on="Energie UV value" class="NumNb (strict)"("Value"=w780) -> ()  [unwired: 2 in, 2 out]
            n430 = property on="Energie UV graph" class="GraphDér (strict)"("Value"=w780) -> ()  [unwired: 2 in, 2 out]
            n431 = property on="valeur de l'horloge en ms" class="NumNb (strict)"() -> ("Value"=w794:u32)  [unwired: 2 in, 2 out]
            n432 = Tick Count (ms)() -> (millisecond timer value=w793:u32)
            n433 = property on="Puissance depolar graph" class="GraphDér (strict)"("Value"=w782) -> ()  [unwired: 2 in, 2 out]
            n434 = property on="Puissance depolar value" class="NumNb (strict)"("Value"=w782) -> ()  [unwired: 2 in, 2 out]
            n435 = Number To Fractional String(number=w780) -> (F-format string=w805:string)  [unwired: 3 in]
            n436 = property on="Energie IR value" class="NumNb (strict)"("Value"=w783) -> ()  [unwired: 2 in, 2 out]
            n437 = property on="Energie IR graph" class="GraphDér (strict)"("Value"=w783) -> ()  [unwired: 2 in, 2 out]
            n438 = Subtract(x=w793, y=w794) -> (x-y=w792:u32)
            n439 = Number To Decimal String(number=w792) -> (decimal integer string=w791:string)  [unwired: 1 in]
            n440 = Concatenate Strings(w795, w796, w791, w796) -> (w790:string)
            n441 = Concatenate Strings(w790, w805, w797) -> (w806:string)
            n442 = Write to Text File(file (use dialog)=w788, text=w806) -> ()  [unwired: 2 in, 3 out]
            n443 = Number To Fractional String(number=w782) -> (F-format string=w803:string)  [unwired: 3 in]
            n444 = property on="Puissance depolar value" class="NumNb (strict)"() -> ("Value"=w819:dbl)  [unwired: 2 in, 2 out]
            n445 = property on="Energie IR value" class="NumNb (strict)"() -> ("Value"=w809:dbl)  [unwired: 2 in, 2 out]
            n446 = Divide(x=w809, y=1000.0) -> (x/y=w807:dbl)
            n447 = Number To Fractional String(number=w783) -> (F-format string=w801:string)  [unwired: 3 in]
            n448 = Concatenate Strings(w790, w803, w797) -> (w804:string)
            n449 = Multiply(x=w807, y=500.0) -> (x*y=w822:dbl)
            n450 = Write to Text File(file (use dialog)=w800, text=w804) -> ()  [unwired: 2 in, 3 out]
            n451 = Concatenate Strings(w790, w801, w797) -> (w802:string)
            n452 = Add(x=w819, y=w822) -> (x+y=w821:dbl)
            n453 = Write to Text File(file (use dialog)=w789, text=w802) -> ()  [unwired: 2 in, 3 out]
            n454 = Divide(x=w819, y=w821) -> (x/y=w818:dbl)
            n455 = Multiply(x=w818, y=100.0) -> (x*y=w813:dbl)
            n456 = property on="Taux depolar value" class="NumNb (strict)"("Value"=w813) -> ()  [unwired: 2 in, 2 out]
            n457 = property on="taux depolar graph" class="GraphDér (strict)"("Value"=w813) -> ()  [unwired: 2 in, 2 out]
            n458 = Greater Or Equal?(x=w813, y=11.0) -> (x >= y?=w811:bool)
            n459 = Less Or Equal?(x=w813, y=9.0) -> (x <= y?=w814:bool)
            n460 = And(x=w814, y=w811) -> (x .and. y?=w812:bool)
            n461 = case shown="Vrai" w814 {
              frame False {
              }
              frame True {
                n462 = property on="Taux depolar indicator" class="BteCoul"("Value"=u32 6618880 ("Boîte de couleur")) -> ()  [unwired: 2 in, 2 out]
              }
            }
            n463 = case shown="Vrai" w812 {
              frame False {
              }
              frame True {
                n464 = property on="Taux depolar indicator" class="BteCoul"("Value"=u32 16755474 ("Boîte de couleur")) -> ()  [unwired: 2 in, 2 out]
              }
            }
            n465 = case shown="Vrai" w811 {
              frame False {
              }
              frame True {
                n466 = property on="Taux depolar indicator" class="BteCoul"("Value"=u32 16711680 ("Boîte de couleur")) -> ()  [unwired: 2 in, 2 out]
              }
            }
            n467 = property on="stop" class="Bool (strict)"() -> ("Value"=w823:bool)  [unwired: 2 in, 2 out]
            n468 = Wait (ms)(milliseconds to wait=u32 1000 ("attente (ms)")) -> ()  [unwired: 1 out]
          }
          n469 = Release Queue(queue=w300, error in (no error)=w299) -> (error out=w304:errorcluster)  [unwired: 1 in, 2 out]
          n470 = Merge Errors(w306, w305, w304) -> (w276:errorcluster)
          n471 = Obtain Queue(name (unnamed)="Energie IR" ("nom (aucun)"), element data type=w282) -> (queue out=w281:refnum<queue>, error out=w280:errorcluster)  [unwired: 3 in, 1 out]
          n472 = property on="COM Port table" class="Tabl (strict)"() -> ("Value"=w287:refnum<visa-resource-name>[])  [unwired: 2 in, 2 out]
          n473 = Bundle(cluster=w282, enum16{"Init", "Read", "Stop", "12sec"}."Init") -> (w279:T3)  [unwired: 1 in]
          n474 = Enqueue Element At Opposite End(queue=w281, element=w279, error in (no error)=w280) -> (queue out=w283:refnum<queue>, error out=w292:errorcluster)  [unwired: 1 in, 1 out]
          n475 = Index Array(array=w287, index=2 ("indice")) -> (element=w271:refnum<visa-resource-name>)
          n476 = while {
            shift-right: [w335] -> w284
            shift-left: w292 -> [w342]
            shift-right: [w334] -> w285
            shift-left: w283 -> [w336]
            shift-right: [w331] -> _
            shift-left: _ -> [w332]
            stop <- w333 stop-if-true
            n477 = Dequeue Element(queue=w336, error in (no error)=w342) -> (queue out=w337:refnum<queue>, element=w341:T3, error out=w338:errorcluster)  [unwired: 1 in, 1 out]
            n478 = Unbundle(w341) -> (w340:enum16{"Init", "Read", "Stop", "12sec"}, "Data"=w339:dbl)
            n479 = case shown="\"Read\"" w340 {
              tunnel: w332 -> [_ w349 w356 w360]
              tunnel: w339 -> [_ w348 w355 _]
              tunnel: w338 -> [w346 w353 w359 w365]
              tunnel: w337 -> [w344 w351 w357 w364]
              tunnel: [w346 w353 w359 w363] -> w335
              tunnel: [FALSE FALSE FALSE TRUE] -> w333
              tunnel: [w344 w351 w357 w361] -> w334
              tunnel: [dbl[] [] dbl[] [] w354 w360] -> w331
              frame "Init", Default {
              }
              frame "12sec" {
                n480 = Insert Into Array(array=w349, new element=w348) -> (w350:dbl[])  [unwired: 1 in]
                n481 = property on="Tableau IR" class="Tabl (strict)"("Value"=w350) -> ()  [unwired: 2 in, 2 out]
              }
              frame "Read" {
                n482 = Insert Into Array(array=w356, new element=w355) -> (w354:dbl[])  [unwired: 1 in]
                n483 = property on="Tableau IR" class="Tabl (strict)"("Value"=w354) -> ()  [unwired: 2 in, 2 out]
              }
              frame "Stop" {
                n484 = Flush Queue(queue=w364, error in (no error)=w365) -> (queue out=w361:refnum<queue>, error out=w363:errorcluster)  [unwired: 1 out]
              }
            }
          }
          n485 = while {
            tunnel: w282 -> [w375]
            shift-right: [w374] -> w290
            shift-left: w292 -> [w373]
            shift-right: [w372] -> _
            shift-left: w283 -> [w376]
            shift-right: [w368] -> w291
            shift-left: w292 -> [w369]
            shift-right: [w366] -> _
            shift-left: w271 -> [w370]
            stop <- w371 stop-if-true
            n486 = event shown="[0] Timeout" {
              selector: _ -> [_ _ _ _ _ _ _ _ _]
              dyn-events: _ -> [_ _ _ _ _ _ _ _ _]
              timeout: 1 -> [_ _ _ _ _ _ _ _ _]
              tunnel: w376 -> [w392 w409 w419 w434 w457 w470 w483 w496 w509]
              tunnel: w375 -> [w391 w408 w422 _ _ _ _ _ _]
              tunnel: [w387 w404 w417 w433 w456 w469 w482 w495 w508] -> w374
              tunnel: w373 -> [w389 w406 w420 w433 w456 w469 w482 w495 w508]
              tunnel: [w388 w405 w421 w434 w457 w470 w483 w496 w509] -> w372
              tunnel: [w386 w403 w416 FALSE w454 w466 w479 w492 w505] -> w371
              tunnel: w370 -> [w377 w394 w412 w428 w451 w462 w475 w488 w501]
              tunnel: w369 -> [w381 w397 w411 w429 w450 w463 w476 w489 w502]
              tunnel: [w380 w396 w411 w425 w449 w461 w474 w487 w500] -> w368
              tunnel: [w378 w395 w412 w426 w448 w460 w473 w486 w499] -> w366
              event Timeout {
                n487 = event-data() -> ()  [unwired: 1 in, 3 out]
                n488 = call "Read Single Value (SubVI).vi"("entrée d'erreur (pas d'erreur)"=w381, "Refnum VISA en entrée"=w377) -> ("sortie d'erreur"=w380:errorcluster, "nombre"=w379:dbl, "Refnum VISA en sortie"=w378:refnum<visa-resource-name>)  [unwired: 6 in, 1 out]
                n489 = Bundle(cluster=w391, enum16{"Init", "Read", "Stop", "12sec"}."Read", "Data"=w379) -> (w390:T3)
                n490 = Enqueue Element(queue=w392, element=w390, error in (no error)=w389) -> (queue out=w388:refnum<queue>, error out=w387:errorcluster)  [unwired: 1 in, 1 out]
                n491 = Unbundle By Name(w387) -> ("status"=w384:bool)
                n492 = Unbundle By Name(w380) -> ("status"=w383:bool)
                n493 = Compound Arithmetic op=OR ("Opérateur arithmétique")(w383, w384, FALSE) -> (w386:bool)
              }
              event "12sec IR": Value Change {
                n494 = event-data() -> ()  [unwired: 1 in, 6 out]
                n495 = call "Read Single Value (SubVI).vi"("entrée d'erreur (pas d'erreur)"=w397, "Refnum VISA en entrée"=w394) -> ("sortie d'erreur"=w396:errorcluster, "nombre"=w393:dbl, "Refnum VISA en sortie"=w395:refnum<visa-resource-name>)  [unwired: 6 in, 1 out]
                n496 = Bundle(cluster=w408, enum16{"Init", "Read", "Stop", "12sec"}."12sec", "Data"=w393) -> (w407:T3)
                n497 = Enqueue Element(queue=w409, element=w407, error in (no error)=w406) -> (queue out=w405:refnum<queue>, error out=w404:errorcluster)  [unwired: 1 in, 1 out]
                n498 = Unbundle By Name(w404) -> ("status"=w401:bool)
                n499 = property on="12sec IR" class="Bool (strict)"("Value"=FALSE ("12sec IR")) -> ()  [unwired: 2 in, 2 out]
                n500 = Unbundle By Name(w396) -> ("status"=w400:bool)
                n501 = Compound Arithmetic op=OR ("Opérateur arithmétique")(w400, w401, FALSE) -> (w403:bool)
              }
              event "stop IR": Value Change {
                n502 = event-data() -> ()  [unwired: 1 in, 6 out]
                n503 = Bundle(cluster=w422, enum16{"Init", "Read", "Stop", "12sec"}."Stop") -> (w418:T3)  [unwired: 1 in]
                n504 = Enqueue Element(queue=w419, element=w418, error in (no error)=w420) -> (queue out=w421:refnum<queue>, error out=w417:errorcluster)  [unwired: 1 in, 1 out]
                n505 = Unbundle By Name(w417) -> ("status"=w414:bool)
                n506 = Unbundle By Name(w411) -> ("status"=w413:bool)
                n507 = Compound Arithmetic op=OR ("Opérateur arithmétique")(w413, w414, TRUE) -> (w416:bool)
              }
              event "Auto Scale (Energie UV)": Value Change {
                w423 = u32 100 ("attente (ms)")
                n508 = event-data() -> ("NewVal"=w431:bool)  [unwired: 1 in, 5 out]
                n509 = call "Wait (SubVI).vi"("error in"=w429, "attente (ms)"=w423) -> ("error out"=w424:errorcluster)  [unwired: 25 in]
                n510 = case shown="Faux" w431 {
                  tunnel: [T2."Enabled" ("Désactivé") T2."Disabled and Grayed Out" ("Désactivé")] -> w430
                  tunnel: w428 -> [w436 w442]
                  tunnel: [w439 w443] -> w426
                  tunnel: w424 -> [w438 w445]
                  tunnel: [w437 w444] -> w427
                  frame False {
                    n511 = call "Port Write (SubVI).vi"("error in"=w438, "write buffer"="*SAS0", "VISA Refnum in"=w436) -> ("error out"=w437:errorcluster, "VISA Refnum out"=w439:refnum<visa-resource-name>)  [unwired: 1 in]
                  }
                  frame True {
                    n512 = call "Port Write (SubVI).vi"("error in"=w445, "write buffer"="*SAS1", "VISA Refnum in"=w442) -> ("error out"=w444:errorcluster, "VISA Refnum out"=w443:refnum<visa-resource-name>)  [unwired: 1 in]
                  }
                }
                n513 = property on="Scale (Watt or Joule) (Energie IR)" class="MDér (strict)"("DisabledEnum"=w430) -> ()  [unwired: 2 in, 2 out]
                n514 = call "Wait (SubVI).vi"("error in"=w427, "attente (ms)"=w423) -> ("error out"=w425:errorcluster)  [unwired: 25 in]
              }
              event "Scale (Watt or Joule) (Energie UV)": Value Change {
                w447 = u32 100 ("attente (ms)")
                n515 = event-data() -> ()  [unwired: 1 in, 6 out]
                n516 = property on="Scale (Watt or Joule) (Energie IR)" class="MDér (strict)"() -> ("Value"=w459:u16)  [unwired: 2 in, 2 out]
                n517 = call "Wait (SubVI).vi"("error in"=w450, "attente (ms)"=w447) -> ("error out"=w455:errorcluster)  [unwired: 25 in]
                n518 = call "Set Scale (SubVI).vi"("error in"=w455, "Scale"=w459, "VISA Refnum in"=w451) -> ("error out"=w458:errorcluster, "VISA Refnum out"=w448:refnum<visa-resource-name>)
                n519 = call "Wait (SubVI).vi"("error in"=w458, "attente (ms)"=w447) -> ("error out"=w449:errorcluster)  [unwired: 25 in]
                n520 = Unbundle By Name(w449) -> ("status"=w453:bool)
                n521 = Compound Arithmetic op=OR ("Opérateur arithmétique")(w453, FALSE) -> (w454:bool)
              }
              event "Trigger Level (% of Scale) (Energie UV)": Value Change {
                w467 = u32 100 ("milliseconds to wait")
                n522 = event-data() -> ()  [unwired: 1 in, 6 out]
                n523 = property on="Trigger Level (% of Scale) (Energie IR)" class="NumNb (strict)"() -> ("Value"=w471:dbl)  [unwired: 2 in, 2 out]
                n524 = call "Wait (SubVI).vi"("error in"=w463, "attente (ms)"=w467) -> ("error out"=w468:errorcluster)  [unwired: 25 in]
                n525 = call "Set Trigger Level (SubVI).vi"("error in"=w468, "Trigger Level (% of Scale)"=w471, "VISA Refnum in"=w462) -> ("error out"=w472:errorcluster, "VISA Refnum out"=w460:refnum<visa-resource-name>)
                n526 = call "Wait (SubVI).vi"("error in"=w472, "attente (ms)"=w467) -> ("error out"=w461:errorcluster)  [unwired: 25 in]
                n527 = Unbundle By Name(w461) -> ("status"=w465:bool)
                n528 = Compound Arithmetic op=OR ("Opérateur arithmétique")(w465, FALSE) -> (w466:bool)
              }
              event "Multiplier (Energie UV)": Value Change {
                w480 = u32 100 ("milliseconds to wait")
                n529 = event-data() -> ()  [unwired: 1 in, 6 out]
                n530 = call "Wait (SubVI).vi"("error in"=w476, "attente (ms)"=w480) -> ("error out"=w481:errorcluster)  [unwired: 25 in]
                n531 = property on="Multiplier (Energie IR)" class="NumNb (strict)"() -> ("Value"=w484:sgl)  [unwired: 2 in, 2 out]
                n532 = call "Set Multiplier (SubVI).vi"("error in"=w481, "Multiplier"=w484, "VISA Refnum in"=w475) -> ("error out"=w485:errorcluster, "VISA Refnum out"=w473:refnum<visa-resource-name>)
                n533 = call "Wait (SubVI).vi"("error in"=w485, "attente (ms)"=w480) -> ("error out"=w474:errorcluster)  [unwired: 25 in]
                n534 = Unbundle By Name(w474) -> ("status"=w477:bool)
                n535 = Compound Arithmetic op=OR ("Opérateur arithmétique")(w477, FALSE) -> (w479:bool)
              }
              event "Offset (Energie UV)": Value Change {
                w493 = u32 100 ("milliseconds to wait")
                n536 = event-data() -> ()  [unwired: 1 in, 6 out]
                n537 = call "Wait (SubVI).vi"("error in"=w489, "attente (ms)"=w493) -> ("error out"=w494:errorcluster)  [unwired: 25 in]
                n538 = property on="Offset (Energie IR)" class="NumNb (strict)"() -> ("Value"=w497:sgl)  [unwired: 2 in, 2 out]
                n539 = call "Set Offset (SubVI).vi"("error in"=w494, "Offset in"=w497, "VISA Refnum in"=w488) -> ("error out"=w498:errorcluster, "VISA Refnum out"=w486:refnum<visa-resource-name>)
                n540 = call "Wait (SubVI).vi"("error in"=w498, "attente (ms)"=w493) -> ("error out"=w487:errorcluster)  [unwired: 25 in]
                n541 = Unbundle By Name(w487) -> ("status"=w490:bool)
                n542 = Compound Arithmetic op=OR ("Opérateur arithmétique")(w490, FALSE) -> (w492:bool)
              }
              event "Wavelength (nm) (Energie UV)": Value Change {
                w506 = u32 100 ("milliseconds to wait")
                n543 = event-data() -> ()  [unwired: 1 in, 6 out]
                n544 = property on="Wavelength (nm) (Energie IR)" class="NumNb (strict)"() -> ("Value"=w510:u32)  [unwired: 2 in, 2 out]
                n545 = call "Wait (SubVI).vi"("error in"=w502, "attente (ms)"=w506) -> ("error out"=w507:errorcluster)  [unwired: 25 in]
                n546 = call "Set Wavelength (SubVI).vi"("error in"=w507, "Wavelength (nm)"=w510, "VISA Refnum in"=w501) -> ("error out"=w511:errorcluster, "VISA Refnum out"=w499:refnum<visa-resource-name>)
                n547 = call "Wait (SubVI).vi"("error in"=w511, "attente (ms)"=w506) -> ("error out"=w500:errorcluster)  [unwired: 25 in]
                n548 = Unbundle By Name(w500) -> ("status"=w503:bool)
                n549 = Compound Arithmetic op=OR ("Opérateur arithmétique")(w503, FALSE) -> (w505:bool)
              }
            }
          }
          n550 = Release Queue(queue=w285, error in (no error)=w284) -> (error out=w289:errorcluster)  [unwired: 1 in, 2 out]
          n551 = Merge Errors(w291, w290, w289) -> (w277:errorcluster)
          n552 = Merge Errors(w277, w276, w275) -> (w274:errorcluster)
        }
        frame Error {
        }
      }
      "sortie d'erreur" <- w269
    }
    frame #2 {
      n553 = property on="sortie d'erreur" class="Clust (strict)"() -> ("Value"=w1016:errorcluster)  [unwired: 2 in, 2 out]
      n554 = case shown="Pas d'erreur" w1016 {
        selector: w1016 -> [_ w1099]
        frame No Error {
          n555 = stacked-sequence {
            frame #0 {
              n556 = property on="Start acquisition" class="Bool (strict)"("Visible"=FALSE) -> ()  [unwired: 2 in, 2 out]
              n557 = property on="stop" class="Bool (strict)"("Visible"=FALSE) -> ()  [unwired: 2 in, 2 out]
              n558 = property on="COM Port table" class="Tabl (strict)"() -> ("Value"=w1018:refnum<visa-resource-name>[])  [unwired: 2 in, 2 out]
              n559 = property on="Commande onglets" class="Onglet (strict)"("DisabledEnum"=T2."Disabled and Grayed Out" ("Désactivé")) -> ()  [unwired: 2 in, 2 out]
              n560 = for {
                tunnel: w1018 -> [w1022] mode=indexing
                n561 = call "Port Close (SubVI).vi"("VISA Refnum in"=w1022) -> ()  [unwired: 1 in, 2 out]
                n562 = Wait (ms)(milliseconds to wait=u32 500 ("attente (ms)")) -> ()  [unwired: 1 out]
              }
              n563 = property on="Update" class="Ch"("Value"="Closing COM Port" ("Étiquette.Texte")) -> ()  [unwired: 2 in, 2 out]
            }
            frame #1 {
              w1024 = enum16{"start", "end", "current"}."end" ("à partir de (0 : start)")
              w1025 = i64 0 ("offset (en octets) (0)")
              n564 = property on="Energie UV file (1sec)" class="Ref (strict)"() -> ("Value"=w1042:refnum<file>)  [unwired: 2 in, 2 out]
              n565 = property on="Energie UV file (stats)" class="Ref (strict)"() -> ("Value"=w1043:refnum<file>)  [unwired: 2 in, 2 out]
              n566 = property on="Puissance depolar file (1sec)" class="Ref (strict)"() -> ("Value"=w1044:refnum<file>)  [unwired: 2 in, 2 out]
              n567 = property on="Puissance depolar file (stats)" class="Ref (strict)"() -> ("Value"=w1045:refnum<file>)  [unwired: 2 in, 2 out]
              n568 = property on="Energie IR file (1sec)" class="Ref (strict)"() -> ("Value"=w1046:refnum<file>)  [unwired: 2 in, 2 out]
              n569 = property on="Energie IR file (stats)" class="Ref (strict)"() -> ("Value"=w1047:refnum<file>)  [unwired: 2 in, 2 out]
              n570 = Get Date/Time In Seconds() -> (seconds since 1Jan1904=w1029:timestamp)
              n571 = Format Date/Time String(time format string (%c)="%d-%m-%Y-%H:%M:%S%3u", seconds (now)=w1029) -> (date/time string=w1027:string)  [unwired: 1 in]
              n572 = Set File Position(offset (in bytes) (0)=w1025, refnum=w1042, from (0:start)=w1024) -> (refnum out=w1035:refnum<file>)  [unwired: 1 in, 1 out]
              n573 = Set File Position(offset (in bytes) (0)=w1025, refnum=w1043, from (0:start)=w1024) -> (refnum out=w1034:refnum<file>)  [unwired: 1 in, 1 out]
              n574 = Set File Position(offset (in bytes) (0)=w1025, refnum=w1044, from (0:start)=w1024) -> (refnum out=w1033:refnum<file>)  [unwired: 1 in, 1 out]
              n575 = Set File Position(offset (in bytes) (0)=w1025, refnum=w1045, from (0:start)=w1024) -> (refnum out=w1032:refnum<file>)  [unwired: 1 in, 1 out]
              n576 = Set File Position(offset (in bytes) (0)=w1025, refnum=w1046, from (0:start)=w1024) -> (refnum out=w1031:refnum<file>)  [unwired: 1 in, 1 out]
              n577 = Set File Position(offset (in bytes) (0)=w1025, refnum=w1047, from (0:start)=w1024) -> (refnum out=w1030:refnum<file>)  [unwired: 1 in, 1 out]
              n578 = Concatenate Strings(w1027) -> (w1026:string)
              n579 = Write to Text File(file (use dialog)=w1035, text=w1026) -> (refnum out=w1041:refnum<file>)  [unwired: 2 in, 2 out]
              n580 = Write to Text File(file (use dialog)=w1034, text=w1026) -> (refnum out=w1040:refnum<file>)  [unwired: 2 in, 2 out]
              n581 = Write to Text File(file (use dialog)=w1033, text=w1026) -> (refnum out=w1039:refnum<file>)  [unwired: 2 in, 2 out]
              n582 = Write to Text File(file (use dialog)=w1032, text=w1026) -> (refnum out=w1038:refnum<file>)  [unwired: 2 in, 2 out]
              n583 = Write to Text File(file (use dialog)=w1031, text=w1026) -> (refnum out=w1037:refnum<file>)  [unwired: 2 in, 2 out]
              n584 = Write to Text File(file (use dialog)=w1030, text=w1026) -> (refnum out=w1036:refnum<file>)  [unwired: 2 in, 2 out]
              n585 = Close File(refnum=w1041) -> ()  [unwired: 1 in, 2 out]
              n586 = Close File(refnum=w1040) -> ()  [unwired: 1 in, 2 out]
              n587 = Close File(refnum=w1039) -> ()  [unwired: 1 in, 2 out]
              n588 = Close File(refnum=w1038) -> ()  [unwired: 1 in, 2 out]
              n589 = Close File(refnum=w1037) -> ()  [unwired: 1 in, 2 out]
              n590 = Close File(refnum=w1036) -> ()  [unwired: 1 in, 2 out]
            }
            frame #2 {
              n591 = stacked-sequence {
                tunnel: [w1066 _ _] -> w1048
                tunnel: [_ w1069 _] -> w1049
                tunnel: [_ _ w1084] -> w1050
                frame #0 {
                  n592 = property on="Auto Scale (Energie UV)" class="Bool (strict)"() -> ("Value"=w1058:bool)  [unwired: 2 in, 2 out]
                  n593 = property on="Multiplier (Energie UV)" class="NumNb (strict)"() -> ("Value"=w1060:sgl)  [unwired: 2 in, 2 out]
                  n594 = property on="Trigger Level (% of Scale) (Energie UV)" class="NumNb (strict)"() -> ("Value"=w1059:dbl)  [unwired: 2 in, 2 out]
                  n595 = property on="COM port (Energie UV)" class="NumNb (strict)"() -> ("Value"=w1065:i64)  [unwired: 2 in, 2 out]
                  n596 = property on="Wavelength (nm) (Energie UV)" class="NumNb (strict)"() -> ("Value"=w1064:u32)  [unwired: 2 in, 2 out]
                  n597 = property on="Offset (Energie UV)" class="NumNb (strict)"() -> ("Value"=w1063:sgl)  [unwired: 2 in, 2 out]
                  n598 = property on="Scale (Watt or Joule) (Energie UV)" class="MDér (strict)"() -> ("Value"=w1055:i32)  [unwired: 2 in, 2 out]
                  n599 = Boolean To (0,1)(Boolean=w1058) -> (0, 1=w1057:i16)
                  n600 = To Double Precision Float(number=w1060) -> (double precision float=w1052:dbl)
                  n601 = To Double Precision Float(number=w1063) -> (double precision float=w1053:dbl)
                  n602 = To Double Precision Float(number=w1057) -> (double precision float=w1056:dbl)
                  n603 = To Double Precision Float(number=w1055) -> (double precision float=w1054:dbl)
                  n604 = To Double Precision Float(number=w1065) -> (double precision float=w1062:dbl)
                  n605 = To Double Precision Float(number=w1064) -> (double precision float=w1061:dbl)
                  n606 = Build Array(w1062, w1061, w1053, w1052, w1059, w1056, w1054) -> (w1066:dbl[])
                }
                frame #1 {
                  n607 = property on="Auto Scale (Puissance depolar)" class="Bool (strict)"() -> ("Value"=w1074:bool)  [unwired: 2 in, 2 out]
                  n608 = property on="Multiplier (Puissance depolar)" class="NumNb (strict)"() -> ("Value"=w1076:sgl)  [unwired: 2 in, 2 out]
                  n609 = property on="Trigger Level (% of Scale) (Puissance depolar)" class="NumNb (strict)"() -> ("Value"=w1075:dbl)  [unwired: 2 in, 2 out]
                  n610 = property on="COM Port (Puissance depolar)" class="NumNb (strict)"() -> ("Value"=w1081:i64)  [unwired: 2 in, 2 out]
                  n611 = property on="Wavelength (nm) (Puissance depolar)" class="NumNb (strict)"() -> ("Value"=w1080:u32)  [unwired: 2 in, 2 out]
                  n612 = property on="Offset (Puissance depolar)" class="NumNb (strict)"() -> ("Value"=w1079:sgl)  [unwired: 2 in, 2 out]
                  n613 = property on="Scale (Watt or Joule) (Puissance depolar)" class="MDér (strict)"() -> ("Value"=w1071:u16)  [unwired: 2 in, 2 out]
                  n614 = Boolean To (0,1)(Boolean=w1074) -> (0, 1=w1073:i16)
                  n615 = To Double Precision Float(number=w1079) -> (double precision float=w1068:dbl)
                  n616 = To Double Precision Float(number=w1076) -> (double precision float=w1067:dbl)
                  n617 = To Double Precision Float(number=w1073) -> (double precision float=w1072:dbl)
                  n618 = To Double Precision Float(number=w1071) -> (double precision float=w1070:dbl)
                  n619 = To Double Precision Float(number=w1081) -> (double precision float=w1078:dbl)
                  n620 = To Double Precision Float(number=w1080) -> (double precision float=w1077:dbl)
                  n621 = Build Array(w1078, w1077, w1068, w1067, w1075, w1072, w1070) -> (w1069:dbl[])
                }
                frame #2 {
                  n622 = property on="Auto Scale (Energie IR)" class="Bool (strict)"() -> ("Value"=w1089:bool)  [unwired: 2 in, 2 out]
                  n623 = property on="Multiplier (Energie IR)" class="NumNb (strict)"() -> ("Value"=w1091:sgl)  [unwired: 2 in, 2 out]
                  n624 = property on="Trigger Level (% of Scale) (Energie IR)" class="NumNb (strict)"() -> ("Value"=w1090:dbl)  [unwired: 2 in, 2 out]
                  n625 = property on="COM Port (Energie IR)" class="NumNb (strict)"() -> ("Value"=w1096:i64)  [unwired: 2 in, 2 out]
                  n626 = property on="Wavelength (nm) (Energie IR)" class="NumNb (strict)"() -> ("Value"=w1095:u32)  [unwired: 2 in, 2 out]
                  n627 = property on="Offset (Energie IR)" class="NumNb (strict)"() -> ("Value"=w1094:sgl)  [unwired: 2 in, 2 out]
                  n628 = property on="Scale (Watt or Joule) (Energie IR)" class="MDér (strict)"() -> ("Value"=w1086:u16)  [unwired: 2 in, 2 out]
                  n629 = Boolean To (0,1)(Boolean=w1089) -> (0, 1=w1088:i16)
                  n630 = To Double Precision Float(number=w1091) -> (double precision float=w1082:dbl)
                  n631 = To Double Precision Float(number=w1094) -> (double precision float=w1083:dbl)
                  n632 = To Double Precision Float(number=w1088) -> (double precision float=w1087:dbl)
                  n633 = To Double Precision Float(number=w1086) -> (double precision float=w1085:dbl)
                  n634 = To Double Precision Float(number=w1096) -> (double precision float=w1093:dbl)
                  n635 = To Double Precision Float(number=w1095) -> (double precision float=w1092:dbl)
                  n636 = Build Array(w1093, w1092, w1083, w1082, w1090, w1087, w1085) -> (w1084:dbl[])
                }
              }
              n637 = property on="file path" class="Chm"() -> ("Value"=w1051:path)  [unwired: 2 in, 2 out]
              n638 = call "Write User File (SubVI).vi"("configuration file path"=w1051, "User file contents Energie UV"=w1048, "User file contents Puissance depolar"=w1049, "User file contents Energie IR"=w1050) -> ()  [unwired: 22 in, 2 out]
            }
            frame #3 {
              n639 = flat-sequence {
                frame #0 {
                  n640 = property on="Update" class="Ch"("Value"="End" ("Étiquette.Texte")) -> ()  [unwired: 2 in, 2 out]
                }
                frame #1 {
                  n641 = Stop(stop? (T)=TRUE ("flag")) -> ()
                }
              }
            }
          }
        }
        frame Error {
          n642 = stacked-sequence {
            tunnel: w1099 -> [_ w1103]
            frame #0 {
              n643 = property on="Start acquisition" class="Bool (strict)"("Visible"=TRUE) -> ()  [unwired: 2 in, 2 out]
              n644 = property on="stop" class="Bool (strict)"("Visible"=FALSE) -> ()  [unwired: 2 in, 2 out]
              n645 = property on="Commande onglets" class="Onglet (strict)"("DisabledEnum"=T2."Enabled" ("Désactivé")) -> ()  [unwired: 2 in, 2 out]
            }
            frame #1 {
              n646 = flat-sequence {
                tunnel: w1103 -> [w1104]
                frame #0 {
                  n647 = call <vilib>:"General Error Handler.vi"("error in (no error)"=w1104) -> ()  [unwired: 10 in, 5 out]
                }
                frame #1 {
                  w1105 = TRUE ("stop ? (V)")
                  n648 = Stop(stop? (T)=w1105) -> ()
                  n649 = Request Deallocation(w1105) -> ()
                }
              }
            }
          }
        }
      }
    }
  }
